vi "运维调试_质控单元.vi"() -> ()   [LabVIEW 2016, in "质控单元.lvlib"]
uses:
  <vilib>/Utility/miscctls.llb/LVPointTypeDef.ctl
  <vilib>/Utility/config.llb/Read Key (I32).vi
  <vilib>/Utility/config.llb/Read Key (Boolean).vi
  <vilib>/Utility/config.llb/Read Key (U32).vi
  <vilib>/Utility/config.llb/Write Key (I32).vi
  <vilib>/Utility/config.llb/Write Key (Boolean).vi
  <vilib>/Utility/config.llb/NI_LVConfig.lvlib
panel:
  out "CODCr母液浓度":dbl caption="加标母液浓度" format="%.2f"
  out "CODCr加标水杯定容体积":dbl caption="加标水杯定容体积" format="%.2f"
  out "CODCr检出限":dbl caption="检出限" format="%.2f"
  out "CODCr量程":dbl caption="量程" format="%.2f"
  out "COD母液浓度":dbl caption="加标母液浓度" format="%.2f"
  out "COD加标水杯定容体积":dbl caption="加标水杯定容体积" format="%.2f"
  out "COD检出限":dbl caption="检出限" format="%.2f"
  out "COD量程":dbl caption="量程" format="%.2f"
  out "总氮母液浓度":dbl caption="加标母液浓度" format="%.3f"
  out "总氮加标水杯定容体积":dbl caption="加标水杯定容体积" format="%.2f"
  out "总氮检出限":dbl caption="检出限" format="%.3f"
  out "总氮量程":dbl caption="量程" format="%.2f"
  out "总磷母液浓度":dbl caption="加标母液浓度" format="%.3f"
  out "总磷加标水杯定容体积":dbl caption="加标水杯定容体积" format="%.2f"
  out "总磷检出限":dbl caption="检出限" format="%.3f"
  out "总磷量程":dbl caption="量程" format="%.2f"
  out "氨氮母液浓度":dbl caption="加标母液浓度" format="%.3f"
  out "氨氮加标水杯定容体积":dbl caption="加标水杯定容体积" format="%.2f"
  out "氨氮检出限":dbl caption="检出限" format="%.3f"
  out "氨氮量程":dbl caption="量程" format="%.2f"
  in  "释放串口":bool
  in  "打开串口":bool
  out "CODCr质控流程中":bool
  out "CODMn质控流程中":bool
  out "总磷质控流程中":bool
  out "总氮质控流程中":bool
  out "氨氮质控流程中":bool
  out "CODCr通讯":bool
  out "CODMn通讯":bool
  out "总磷总氮通讯":bool
  out "氨氮通讯":bool
  out "CODCr传感器状态显示":bool
  out "CODCr超时报警":bool
  out "CODMn超时报警":bool
  out "总磷总氮超时报警":bool
  out "氨氮进样超时报警":bool
  out "CODMn传感器状态显示":bool
  out "总磷总氮传感器状态显示":bool
  out "氨氮传感器状态显示":bool
  out "CODCr流程中断报警":bool
  out "总磷总氮流程中断报警":bool
  out "CODMn流程中断报警":bool
  out "氨氮流程中断报警":bool
  in  "手动调试":bool
  in  "报警清除":bool
  in  "查看":bool
  in  "停止测量":bool
  in  "加标回收":bool
  in  "平行样测试":bool
  in  "CODCr量程选择":enum32{"H", "L", "AUTO"}(ring)
  in  "CODCr选择":bool
  out "CODCr加标回收率":dbl caption="加标回收率" format="%.2f"
  out "CODCr加标体积":dbl caption="加标体积" format="%.3f"
  out "CODCr加标后水样浓度":dbl caption="加标后水样浓度" format="%.2f"
  out "CODCr加标前水样浓度":dbl caption="加标前水样浓度" format="%.2f"
  out "CODCr状态":u16(ring) caption="状态" items=["待机", "润洗", "进样", "等待取液", "排液"]
  out "质控流程中":bool
  in  "CODMn量程选择":enum32{"H", "L", "AUTO"}(ring)
  in  "总磷量程选择":enum32{"H", "L", "AUTO"}(ring)=enum."AUTO"
  in  "总氮量程选择":enum32{"H", "L", "AUTO"}(ring)=enum."AUTO"
  in  "氨氮量程选择":enum32{"H", "L", "AUTO"}(ring)=enum."AUTO"
  in  "CODMn选择":bool
  in  "总磷总氮模块选择":bool
  in  "氨氮模块":bool
  in  "背隙补偿步数 3":i32 min=0 max=2000
  in  "背隙补偿步数 2":i32 min=0 max=2000
  in  "背隙补偿步数":i32 min=0 max=2000
  out "总氮加标回收率":dbl caption="加标回收率" format="%.2f"
  out "总氮加标体积":dbl caption="加标体积" format="%.3f"
  out "总氮加标后水样浓度":dbl caption="加标后水样浓度" format="%.3f"
  out "总氮加标前水样浓度":dbl caption="加标前水样浓度" format="%.3f"
  out "总氮状态":u16(ring) caption="状态" items=["待机", "润洗", "进样", "等待取液", "排液"]
  in  "返回":bool
  out "COD加标回收率":dbl caption="加标回收率" format="%.2f"
  out "COD加标体积":dbl caption="加标体积" format="%.3f"
  out "COD加标后水样浓度":dbl caption="加标后水样浓度" format="%.2f"
  out "COD加标前水样浓度":dbl caption="加标前水样浓度" format="%.2f"
  out "CODMn状态":u16(ring) caption="状态" items=["待机", "润洗", "进样", "等待取液", "排液"]
  out "总磷加标回收率":dbl caption="加标回收率" format="%.2f"
  out "总磷加标体积":dbl caption="加标体积" format="%.3f"
  out "总磷加标后水样浓度":dbl caption="加标后水样浓度" format="%.3f"
  out "总磷加标前水样浓度":dbl caption="加标前水样浓度" format="%.3f"
  out "总磷状态":u16(ring) caption="状态" items=["待机", "润洗", "进样", "等待取液", "排液"]
  out "氨氮加标回收率":dbl caption="加标回收率" format="%.2f"
  out "氨氮加标体积":dbl caption="加标体积" format="%.3f"
  out "氨氮加标后水样浓度":dbl caption="加标后水样浓度" format="%.3f"
  out "氨氮加标前水样浓度":dbl caption="加标前水样浓度" format="%.3f"
  out "氨氮状态":u16(ring) caption="状态" items=["待机", "润洗", "进样", "等待取液", "排液"]
  # "氨氮"
  # "总磷"
  # "总氮"
  # "CODMn"
  # "CODCr"
  # "参数配置区"
  # "2000步等于1mL\n100步等于0.05mL\n20步等于0.01mL\n2步等于0.001mL\n（初始默认100步）"
  # "CODCr质控参数"
  # "mg/L"
  # "mL"
  # "mg/L"
  # "mg/L"
  # "CODMn质控参数"
  # "mg/L"
  # "mL"
  # "mg/L"
  # "mg/L"
  # "总氮质控参数"
  # "mg/L"
  # "mL"
  # "mg/L"
  # "mg/L"
  # "总磷质控参数"
  # "mg/L"
  # "mL"
  # "mg/L"
  # "mg/L"
  # "氨氮质控参数"
  # "mg/L"
  # "mL"
  # "mg/L"
  # "mg/L"
  # "%"
  # "mL"
  # "mg/L"
  # "mg/L"
  # "%"
  # "mL"
  # "mg/L"
  # "mg/L"
  # "%"
  # "mL"
  # "mg/L"
  # "mg/L"
  # "%"
  # "mL"
  # "mg/L"
  # "mg/L"
  # "%"
  # "mL"
  # "mg/L"
  # "mg/L"
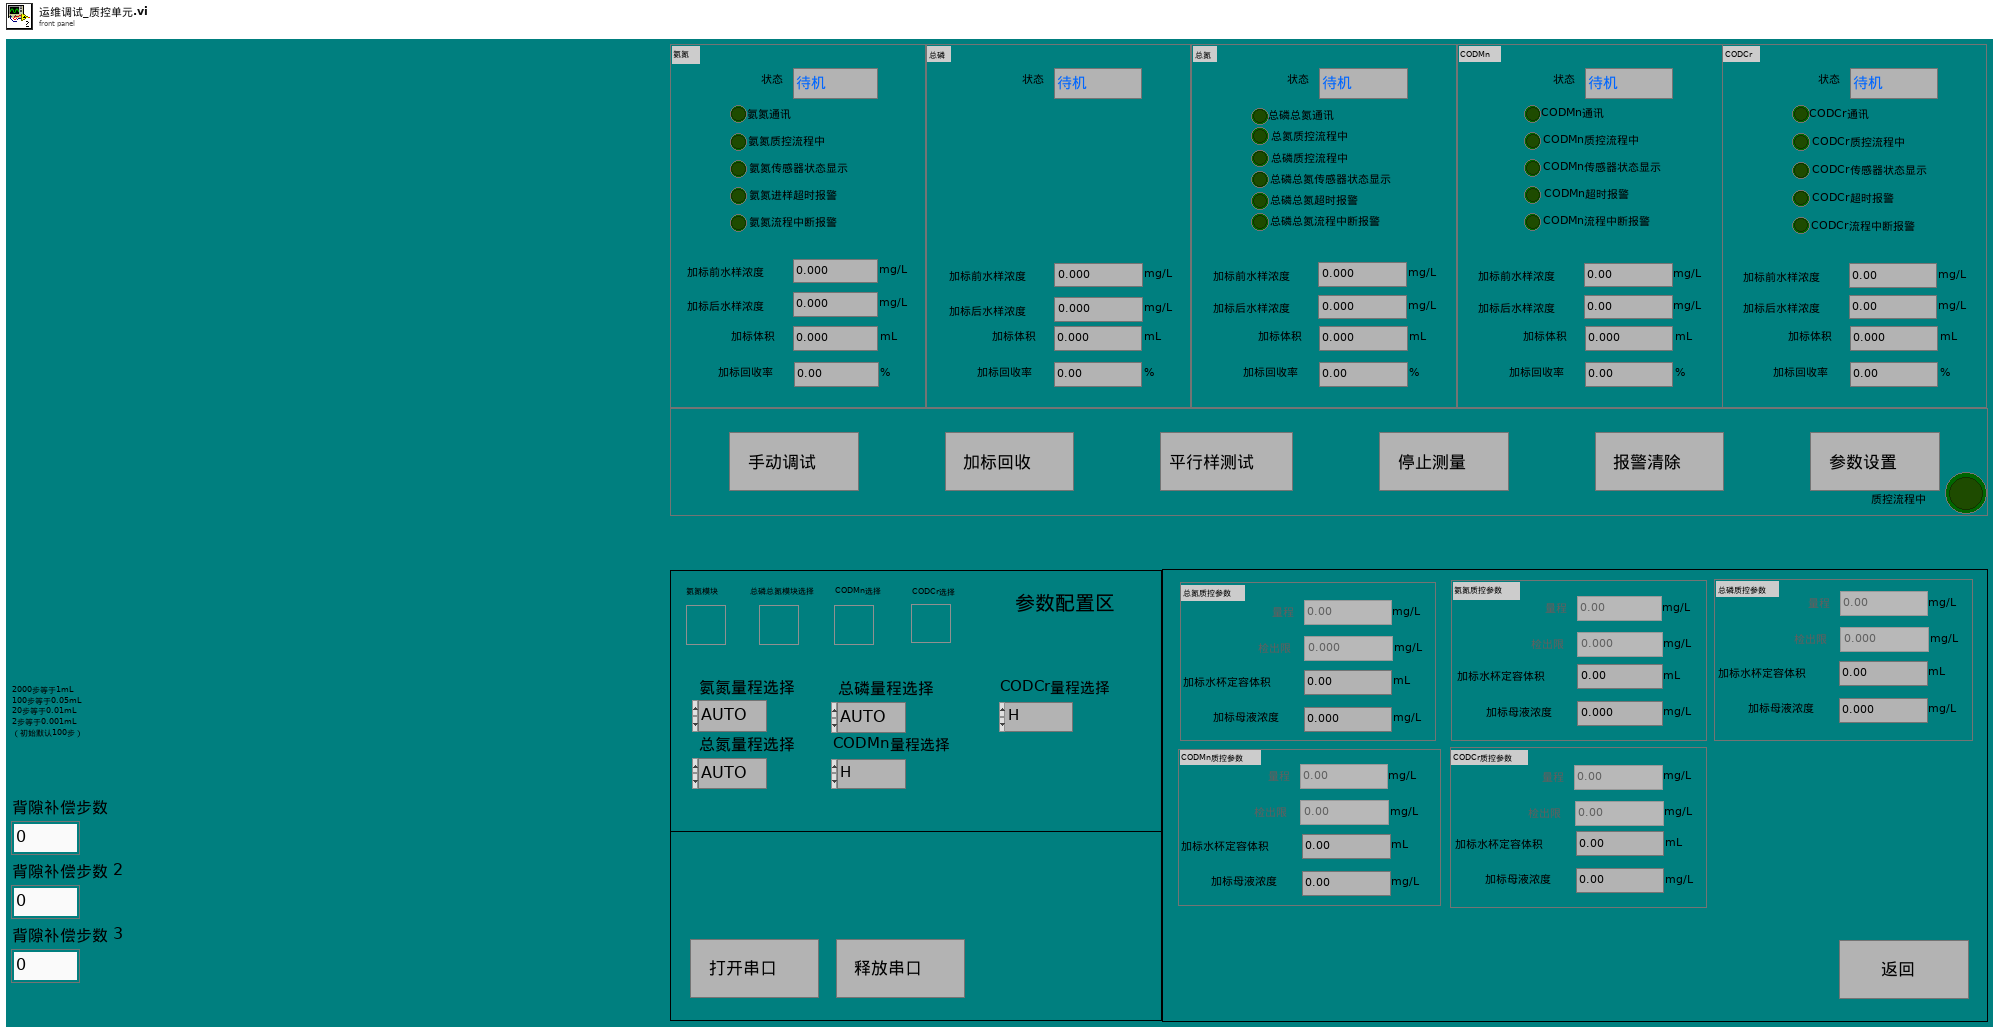
[diagram p1: front panel]
types:
  T1 = typedef "LVPointTypeDef.ctl" = cluster{"Horizontal":i16, "Vertical":i16}
  T2 = typedef "NI_LVConfig.lvlib/Config Data RefNum.ctl" = refnum<k1>
  T3 = cluster{"量程":dbl, "检出限":dbl, "加标前水样浓度":dbl, "加标后水样浓度":dbl, "加标水杯定容体积":dbl, "加标母液浓度":dbl, "加标体积":dbl, "加标回收率":dbl}
  T4 = enum8{"Enabled", "Disabled", "Disabled and Grayed Out"}
  T5 = cluster{"是否启用仪器":bool, "CODMn":cluster{"启动测量模式":cluster{"测量模式":enum16{"水样测量", "标样核查", "加标回收", "平行样", "校零", "校标"}}, "确定按钮":bool}, "启动模块":cluster{"氨氮":bool, "总磷":bool, "总氮":bool, "CODMn":bool, "CODCr":bool}, "常规启动":bool, "直接启动":bool}
  T6 = cluster{"参数启用":cluster{"CODMn":bool, "总磷":bool, "总氮":bool, "氨氮":bool, "CODcr":bool}, "采配水是否启动":bool}
  T7 = cluster{"命令":string, cluster{"starting address":u16, "holding register value":u16}}
  T8 = cluster{"氨氮":bool, "总磷":bool, "总氮":bool, "CODMn":bool, "CODCr":bool}
  T9 = enum32{"Bad", "Idle", "Run top level", "Running"}
  T10 = cluster{"CODMn":bool, "总磷":bool, "总氮":bool, "氨氮":bool, "CODCr":bool}
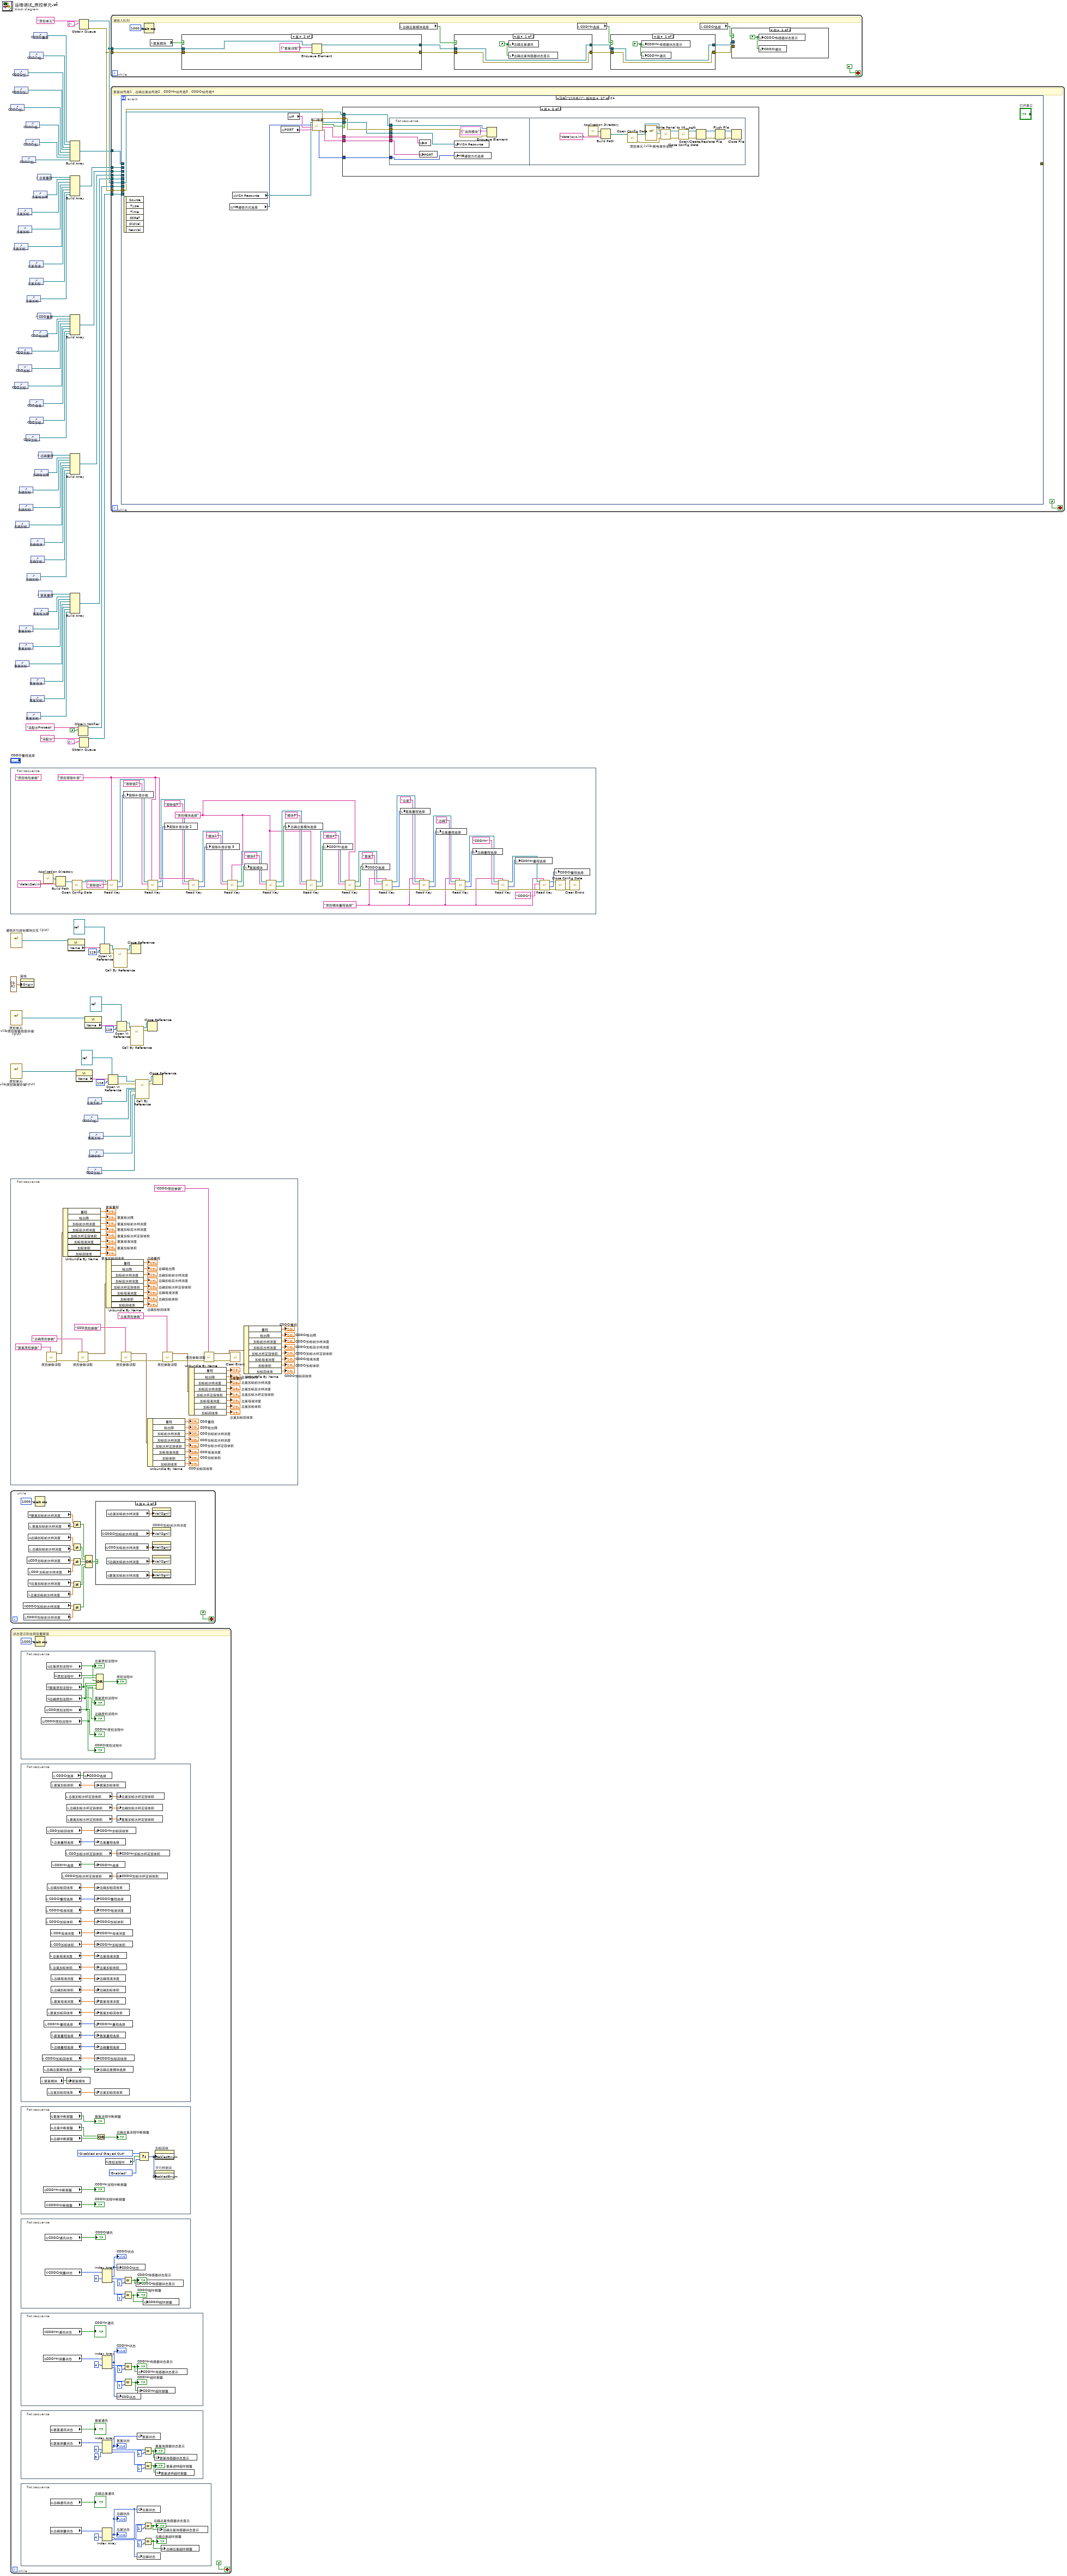
[diagram p0: block diagram]
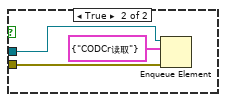
[diagram p2: hidden frame]
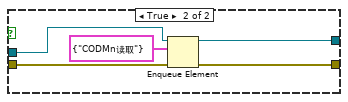
[diagram p3: hidden frame]
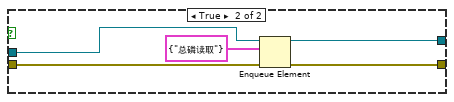
[diagram p4: hidden frame]
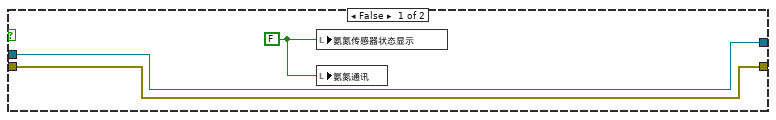
[diagram p5: hidden frame]
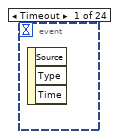
[diagram p7: hidden frame]
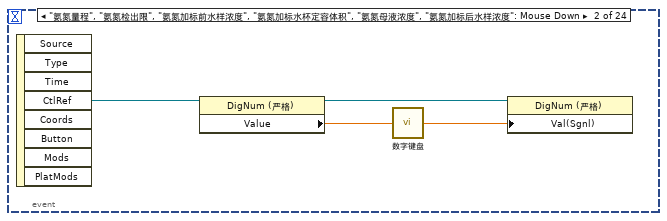
[diagram p8: hidden frame]
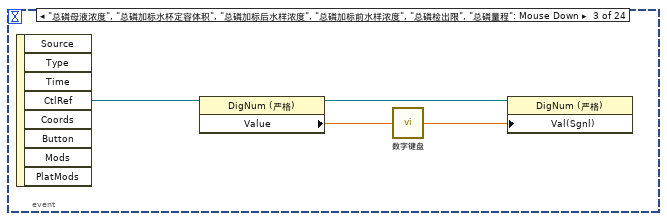
[diagram p9: hidden frame]
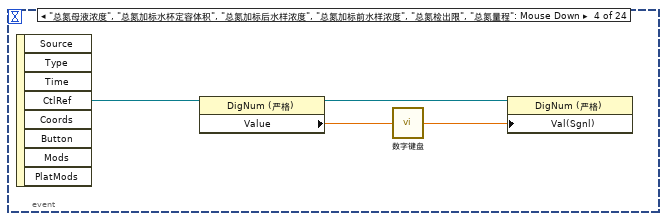
[diagram p10: hidden frame]
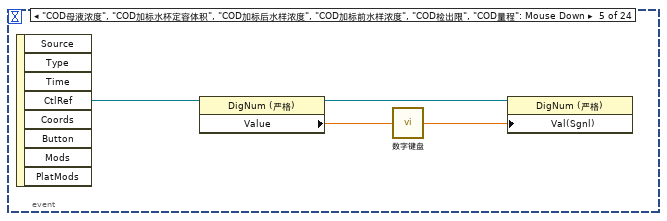
[diagram p11: hidden frame]
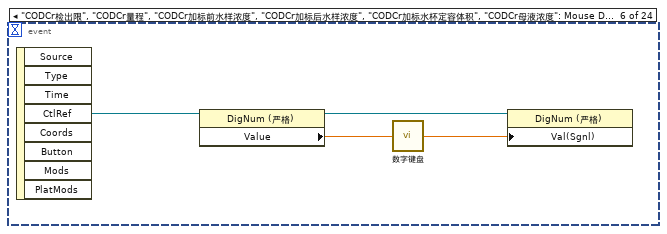
[diagram p12: hidden frame]
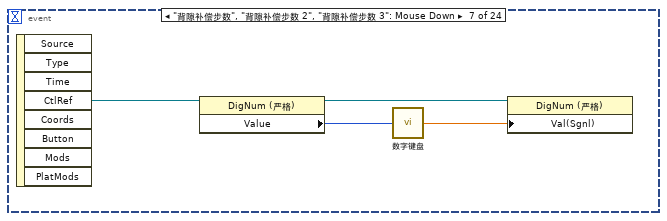
[diagram p13: hidden frame]
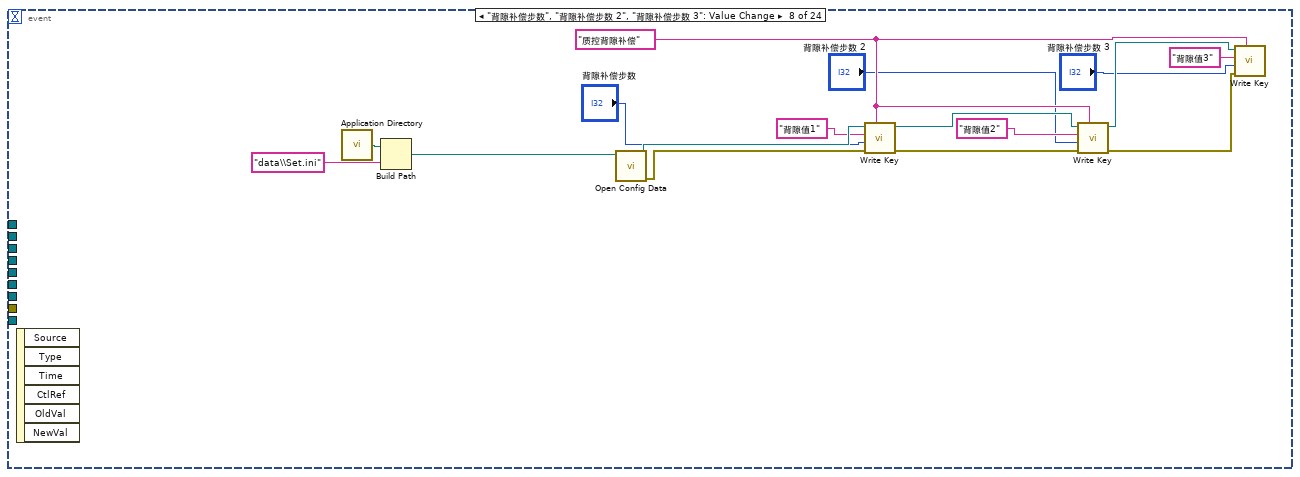
[diagram p14: hidden frame]
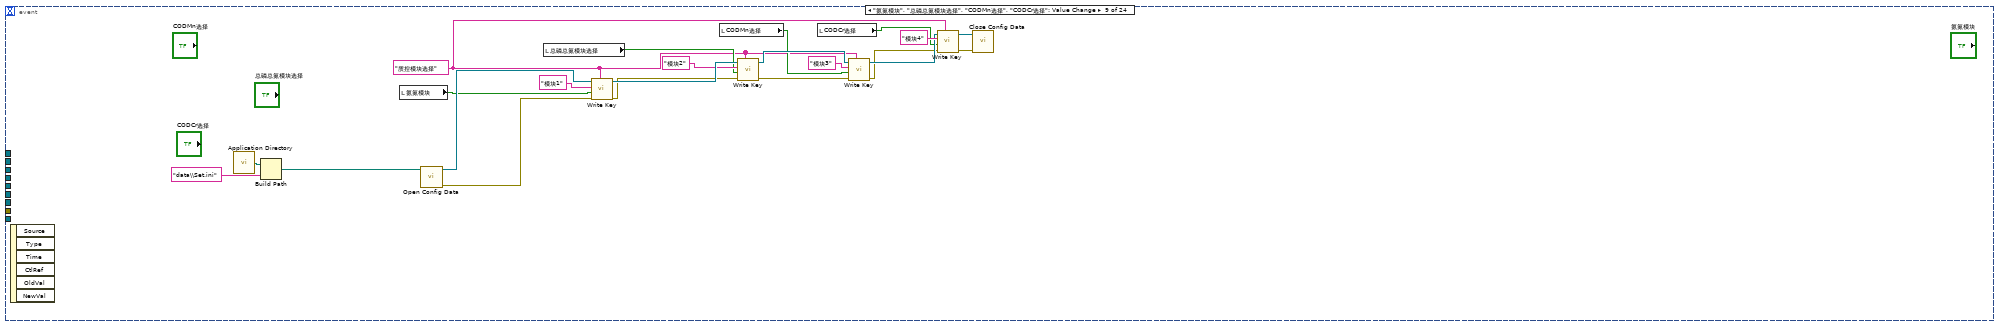
[diagram p15: hidden frame]
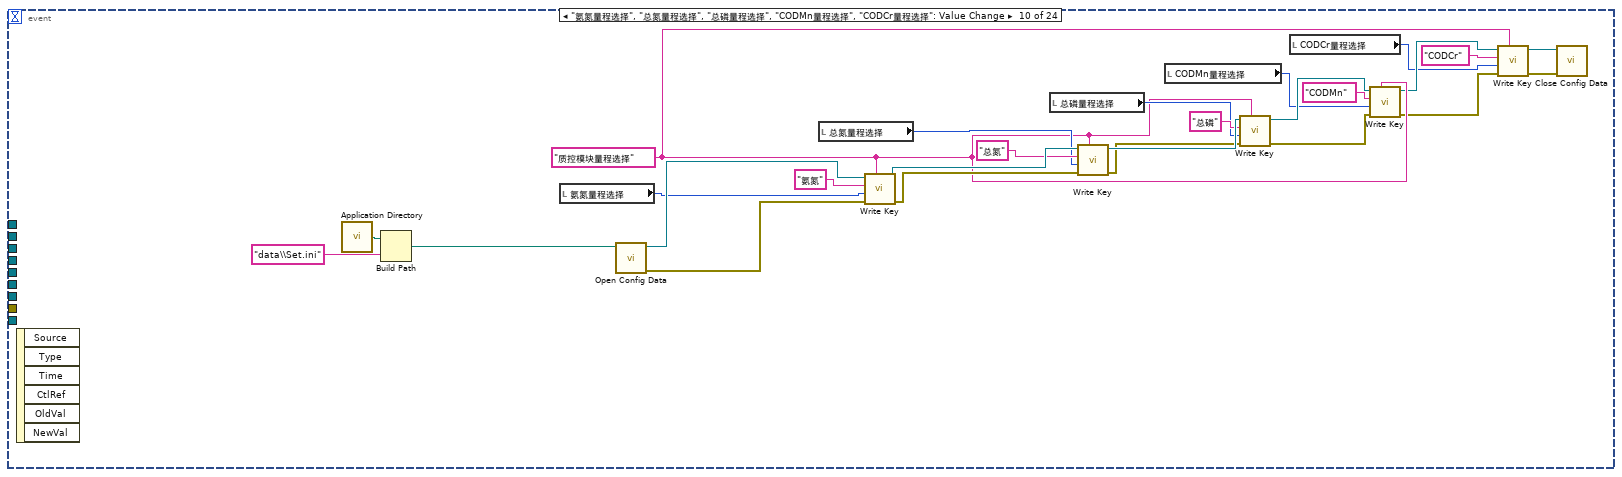
[diagram p16: hidden frame]
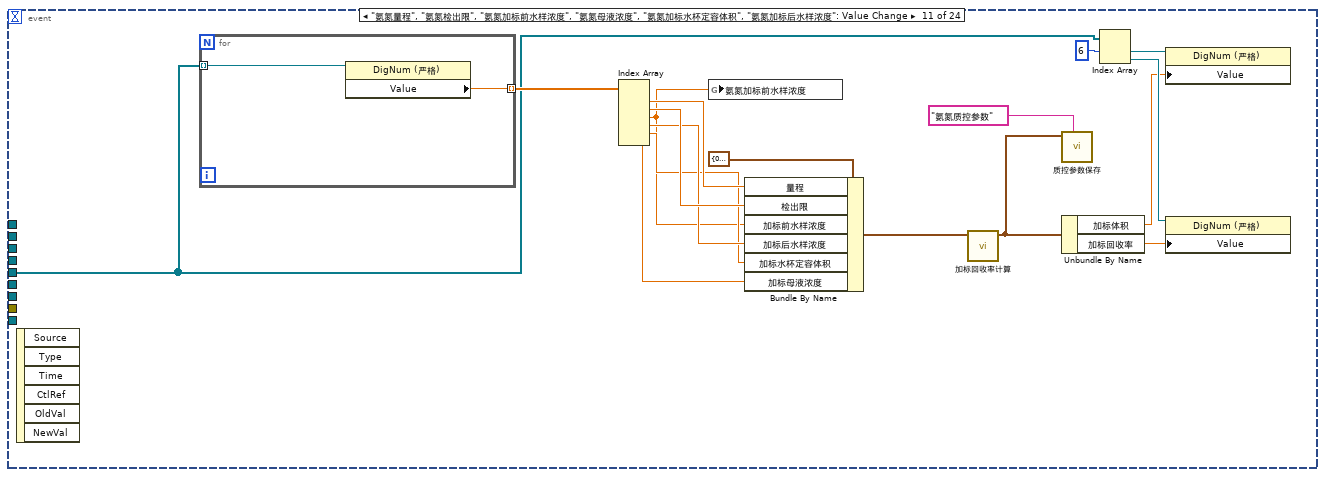
[diagram p17: hidden frame]
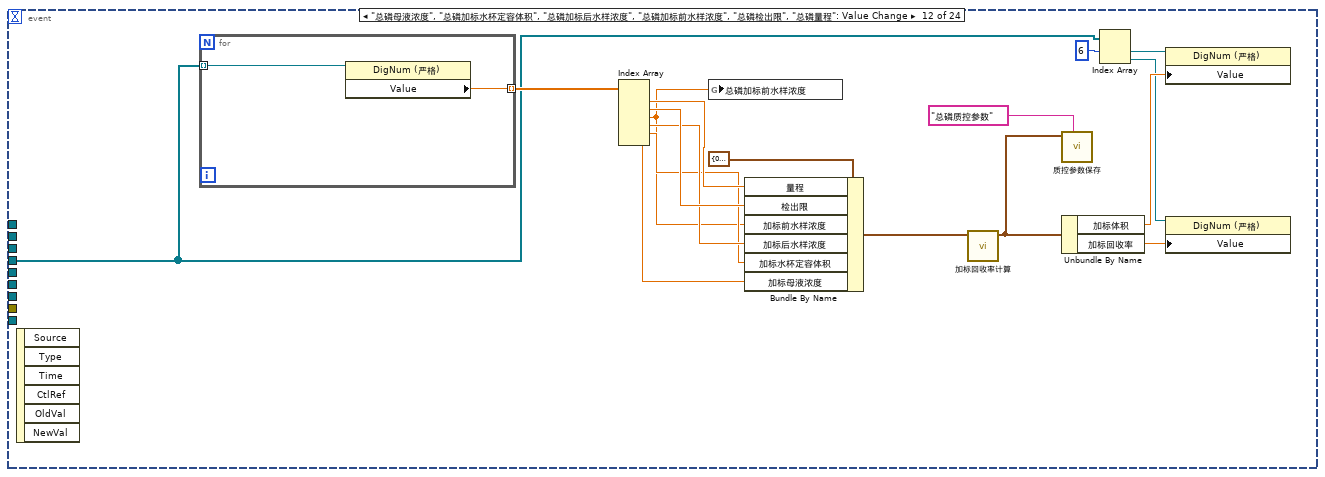
[diagram p18: hidden frame]
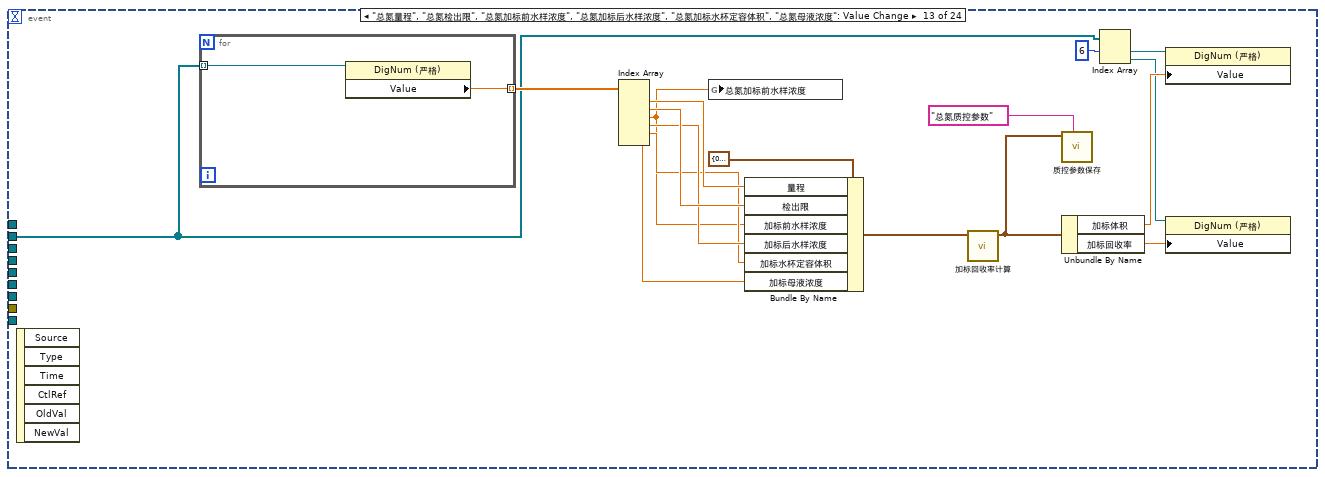
[diagram p19: hidden frame]
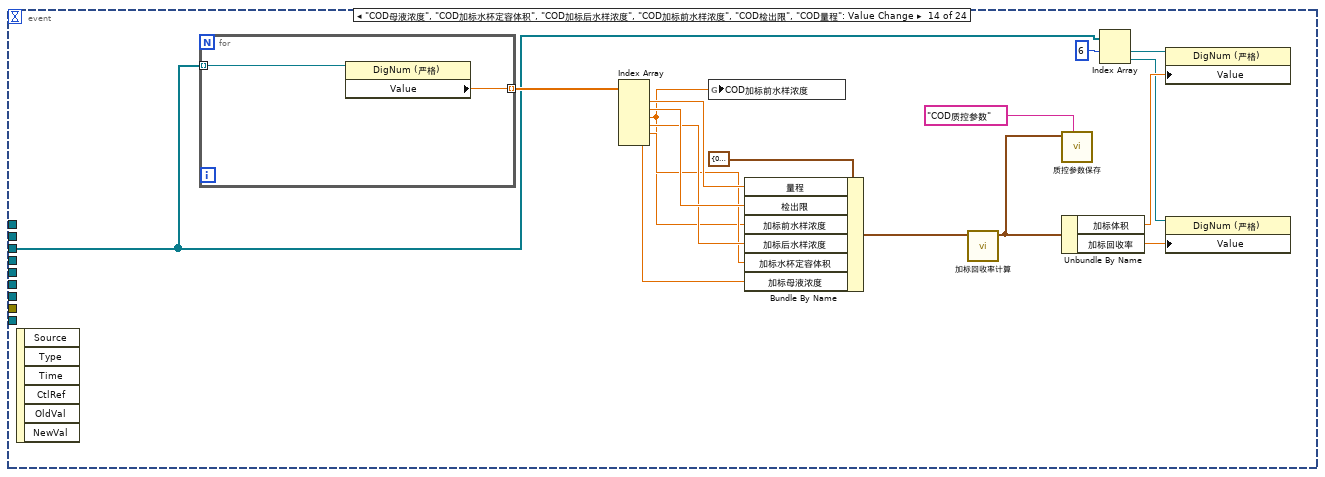
[diagram p20: hidden frame]
diagram:
  n1 = control-ref of="CODCr加标水杯定容体积"() -> (w38:refnum<vi>)
  n2 = flat-sequence {
    frame #0 {
      w100 = "质控模块量程选择" ("section")
      w92 = "质控模块选择" ("section")
      (unwired) "质控线性参数" ("section")
      w136 = "质控背隙补偿" ("section")
      n3 = call <vilib>:"Application Directory.vi"() -> ("Application Directory"=w142:path)
      n4 = Build Path(base path=w142, name or relative path="data\\Set.ini" ("名称或相对路径")) -> (appended path=w140:path)
      n5 = call <vilib>:"Open Config Data.vi"("configuration file path"=w140) -> ("error out"=w138:errorcluster, "refnum"=w139:T2)  [unwired: 8 in, 1 out]
      n6 = call-poly <vilib>:"Read Key.vi"("section"=w136, "error in (no error)"=w138, "key"="背隙值1", "refnum"=w139) -> ("error out"=w133:errorcluster, "value"=w128:i32, "refnum out"=w135:T2)  [unwired: 4 in, 1 out]
      n7 = local write "背隙补偿步数"(w128) -> ()
      n8 = call-poly <vilib>:"Read Key.vi"("section"=w136, "error in (no error)"=w133, "key"="背隙值2", "refnum"=w135) -> ("error out"=w131:errorcluster, "value"=w129:i32, "refnum out"=w132:T2)  [unwired: 4 in, 1 out]
      n9 = local write "背隙补偿步数 2"(w129) -> ()
      n10 = call-poly <vilib>:"Read Key.vi"("section"=w136, "error in (no error)"=w131, "key"="背隙值3", "refnum"=w132) -> ("error out"=w87:errorcluster, "value"=w127:i32, "refnum out"=w88:T2)  [unwired: 4 in, 1 out]
      n11 = local write "背隙补偿步数 3"(w127) -> ()
      n12 = call-poly <vilib>:"Read Key.vi"("section"=w92, "error in (no error)"=w87, "key"="模块1" ("section"), "refnum"=w88) -> ("error out"=w125:errorcluster, "value"=w117:bool, "refnum out"=w126:T2)  [unwired: 4 in, 1 out]
      n13 = local write "氨氮模块"(w117) -> ()
      n14 = call-poly <vilib>:"Read Key.vi"("section"=w92, "error in (no error)"=w125, "key"="模块2" ("section"), "refnum"=w126) -> ("error out"=w123:errorcluster, "value"=w118:bool, "refnum out"=w124:T2)  [unwired: 4 in, 1 out]
      n15 = local write "总磷总氮模块选择"(w118) -> ()
      n16 = call-poly <vilib>:"Read Key.vi"("section"=w92, "error in (no error)"=w123, "key"="模块3" ("section"), "refnum"=w124) -> ("error out"=w94:errorcluster, "value"=w119:bool, "refnum out"=w95:T2)  [unwired: 4 in, 1 out]
      n17 = local write "CODMn选择"(w119) -> ()
      n18 = call-poly <vilib>:"Read Key.vi"("section"=w92, "error in (no error)"=w94, "key"="模块4", "refnum"=w95) -> ("error out"=w90:errorcluster, "value"=w89:bool, "refnum out"=w91:T2)  [unwired: 4 in, 1 out]
      n19 = local write "CODCr选择"(w89) -> ()
      n20 = call-poly <vilib>:"Read Key.vi"("section"=w100, "error in (no error)"=w90, "key"="氨氮" ("section"), "refnum"=w91) -> ("error out"=w115:errorcluster, "value"=w106:u32, "refnum out"=w116:T2)  [unwired: 4 in, 1 out]
      n21 = local write "氨氮量程选择"(w106) -> ()
      n22 = call-poly <vilib>:"Read Key.vi"("section"=w100, "error in (no error)"=w115, "key"="总氮" ("section"), "refnum"=w116) -> ("error out"=w113:errorcluster, "value"=w105:u32, "refnum out"=w114:T2)  [unwired: 4 in, 1 out]
      n23 = local write "总氮量程选择"(w105) -> ()
      n24 = call-poly <vilib>:"Read Key.vi"("section"=w100, "error in (no error)"=w113, "key"="总磷" ("section"), "refnum"=w114) -> ("error out"=w111:errorcluster, "value"=w104:u32, "refnum out"=w112:T2)  [unwired: 4 in, 1 out]
      n25 = local write "总磷量程选择"(w104) -> ()
      n26 = call-poly <vilib>:"Read Key.vi"("section"=w100, "error in (no error)"=w111, "key"="CODMn" ("section"), "refnum"=w112) -> ("error out"=w101:errorcluster, "value"=w103:u32, "refnum out"=w102:T2)  [unwired: 4 in, 1 out]
      n27 = local write "CODMn量程选择"(w103) -> ()
      n28 = call-poly <vilib>:"Read Key.vi"("section"=w100, "error in (no error)"=w101, "key"="CODCr" ("section"), "refnum"=w102) -> ("error out"=w97:errorcluster, "value"=w98:u32, "refnum out"=w96:T2)  [unwired: 4 in, 1 out]
      n29 = local write "CODCr量程选择"(w98) -> ()
      n30 = call <vilib>:"Close Config Data.vi"("error in (no error)"=w97, "refnum"=w96) -> ("error out"=w86:errorcluster)  [unwired: 8 in, 1 out]
      n31 = call <vilib>:"Clear Errors.vi"("error in (no error)"=w86) -> ()  [unwired: 5 in, 2 out]
    }
  }
  n32 = vi-ref "通信并与其他模块交互 (子VI).vi"() -> (w26:refnum<vi>)
  n33 = vi-ref "质控单元.lvlib:质控报警信息存储 (子VI).vi"() -> (w21:refnum<vi>)
  n34 = vi-ref "质控单元.lvlib:质控数据存储(子VI).vi"() -> (w6:refnum<vi>)
  n35 = flat-sequence {
    frame #0 {
      n36 = call "质控参数读取.vi"("section"="氨氮质控参数") -> ("error out"=w177:errorcluster, "参数"=w196:T3)  [unwired: 9 in]
      n37 = Unbundle By Name(w196) -> ("量程"=→"氨氮量程":dbl, "检出限"=→"氨氮检出限":dbl, "加标前水样浓度"=→"氨氮加标前水样浓度":dbl, "加标后水样浓度"=→"氨氮加标后水样浓度":dbl, "加标水杯定容体积"=→"氨氮加标水杯定容体积":dbl, "加标母液浓度"=→"氨氮母液浓度":dbl, "加标体积"=→"氨氮加标体积":dbl, "加标回收率"=→"氨氮加标回收率":dbl)
      n38 = call "质控参数读取.vi"("section"="总磷质控参数", "error in (no error)"=w177) -> ("error out"=w174:errorcluster, "参数"=w186:T3)  [unwired: 8 in]
      n39 = Unbundle By Name(w186) -> ("量程"=→"总磷量程":dbl, "检出限"=→"总磷检出限":dbl, "加标前水样浓度"=→"总磷加标前水样浓度":dbl, "加标后水样浓度"=→"总磷加标后水样浓度":dbl, "加标水杯定容体积"=→"总磷加标水杯定容体积":dbl, "加标母液浓度"=→"总磷母液浓度":dbl, "加标体积"=→"总磷加标体积":dbl, "加标回收率"=→"总磷加标回收率":dbl)
      n40 = call "质控参数读取.vi"("section"="COD质控参数", "error in (no error)"=w174) -> ("error out"=w164:errorcluster, "参数"=w176:T3)  [unwired: 8 in]
      n41 = Unbundle By Name(w176) -> ("量程"=→"COD量程":dbl, "检出限"=→"COD检出限":dbl, "加标前水样浓度"=→"COD加标前水样浓度":dbl, "加标后水样浓度"=→"COD加标后水样浓度":dbl, "加标水杯定容体积"=→"COD加标水杯定容体积":dbl, "加标母液浓度"=→"COD母液浓度":dbl, "加标体积"=→"COD加标体积":dbl, "加标回收率"=→"COD加标回收率":dbl)
      n42 = call "质控参数读取.vi"("section"="总氮质控参数", "error in (no error)"=w164) -> ("error out"=w152:errorcluster, "参数"=w163:T3)  [unwired: 8 in]
      n43 = Unbundle By Name(w163) -> ("量程"=→"总氮量程":dbl, "检出限"=→"总氮检出限":dbl, "加标前水样浓度"=→"总氮加标前水样浓度":dbl, "加标后水样浓度"=→"总氮加标后水样浓度":dbl, "加标水杯定容体积"=→"总氮加标水杯定容体积":dbl, "加标母液浓度"=→"总氮母液浓度":dbl, "加标体积"=→"总氮加标体积":dbl, "加标回收率"=→"总氮加标回收率":dbl)
      n44 = call "质控参数读取.vi"("section"="CODCr质控参数", "error in (no error)"=w152) -> ("error out"=w143:errorcluster, "参数"=w153:T3)  [unwired: 8 in]
      n45 = call <vilib>:"Clear Errors.vi"("error in (no error)"=w143) -> ()  [unwired: 5 in, 2 out]
      n46 = Unbundle By Name(w153) -> ("量程"=→"CODCr量程":dbl, "检出限"=→"CODCr检出限":dbl, "加标前水样浓度"=→"CODCr加标前水样浓度":dbl, "加标后水样浓度"=→"CODCr加标后水样浓度":dbl, "加标水杯定容体积"=→"CODCr加标水杯定容体积":dbl, "加标母液浓度"=→"CODCr母液浓度":dbl, "加标体积"=→"CODCr加标体积":dbl, "加标回收率"=→"CODCr加标回收率":dbl)
    }
  }
  n47 = while {
    stop <- FALSE stop-if-true
    n48 = global read "水样浓度全局.vi" "CODCr加标前水样浓度"() -> (w200:dbl)
    n49 = local read "CODCr加标前水样浓度"() -> (w199:dbl)
    n50 = global read "水样浓度全局.vi" "COD加标前水样浓度"() -> (w209:dbl)
    n51 = local read "总氮加标前水样浓度"() -> (w203:dbl)
    n52 = global read "水样浓度全局.vi" "氨氮加标前水样浓度"() -> (w213:dbl)
    n53 = global read "水样浓度全局.vi" "总磷加标前水样浓度"() -> (w211:dbl)
    n54 = local read "COD加标前水样浓度"() -> (w208:dbl)
    n55 = global read "水样浓度全局.vi" "总氮加标前水样浓度"() -> (w202:dbl)
    n56 = local read "氨氮加标前水样浓度"() -> (w212:dbl)
    n57 = local read "总磷加标前水样浓度"() -> (w210:dbl)
    n58 = Wait (ms)(milliseconds to wait=u32 1000 ("等待时间（毫秒）")) -> ()  [unwired: 1 out]
    n59 = Not Equal?(x=w213, y=w212) -> (x != y?=w207:bool)
    n60 = Not Equal?(x=w211, y=w210) -> (x != y?=w205:bool)
    n61 = Not Equal?(x=w209, y=w208) -> (x != y?=w204:bool)
    n62 = Not Equal?(x=w202, y=w203) -> (x != y?=w201:bool)
    n63 = Not Equal?(x=w200, y=w199) -> (x != y?=w198:bool)
    n64 = Compound Arithmetic op=OR ("复合运算")(w207, w205, w204, w201, w198) -> (w206:bool)
    n65 = case shown="真" w206 {
      frame False {
      }
      frame True {
        n66 = global read "水样浓度全局.vi" "CODCr加标前水样浓度"() -> (w216:dbl)
        n67 = global read "水样浓度全局.vi" "COD加标前水样浓度"() -> (w218:dbl)
        n68 = global read "水样浓度全局.vi" "总氮加标前水样浓度"() -> (w217:dbl)
        n69 = global read "水样浓度全局.vi" "总磷加标前水样浓度"() -> (w219:dbl)
        n70 = global read "水样浓度全局.vi" "氨氮加标前水样浓度"() -> (w220:dbl)
        n71 = property on="总氮加标前水样浓度" class="DigNum (严格)"("Val(Sgnl)"=w217) -> ()  [unwired: 2 in, 2 out]
        n72 = property on="CODCr加标前水样浓度" class="DigNum (严格)"("Val(Sgnl)"=w216) -> ()  [unwired: 2 in, 2 out]
        n73 = property on="COD加标前水样浓度" class="DigNum (严格)"("Val(Sgnl)"=w218) -> ()  [unwired: 2 in, 2 out]
        n74 = property on="总磷加标前水样浓度" class="DigNum (严格)"("Val(Sgnl)"=w219) -> ()  [unwired: 2 in, 2 out]
        n75 = property on="氨氮加标前水样浓度" class="DigNum (严格)"("Val(Sgnl)"=w220) -> ()  [unwired: 2 in, 2 out]
      }
    }
  }
  n76 = while {
    stop <- FALSE stop-if-true
    # "状态显示和全局变量赋值"
    n77 = flat-sequence {
      frame #0 {
        n78 = global read "质控测完标志全局 1.vi" "CODCr质控流程中"() -> (w303:bool)
        "CODCr质控流程中" <- w303
        n79 = global read "质控测完标志全局 1.vi" "COD质控流程中"() -> (w304:bool)
        "CODMn质控流程中" <- w304
        n80 = global read "质控测完标志全局 1.vi" "总氮质控流程中"() -> (w306:bool)
        "总氮质控流程中" <- w306
        n81 = global read "质控测完标志全局 1.vi" "氨氮质控流程中"() -> (w307:bool)
        "氨氮质控流程中" <- w307
        n82 = global read "质控测完标志全局 1.vi" "总磷质控流程中"() -> (w305:bool)
        "总磷质控流程中" <- w305
        n83 = global read "质控测完标志全局 1.vi" "质控流程中"() -> (w309:bool)
        n84 = Compound Arithmetic op=OR ("复合运算")(w309, w307, w306, w305, w304, w303) -> (→"质控流程中":bool)
      }
    }
    n85 = flat-sequence {
      frame #0 {
        n86 = local read "氨氮模块"() -> (w297:bool)
        n87 = local read "CODCr加标回收率"() -> (w278:dbl)
        n88 = local read "总磷总氮模块选择"() -> (w296:bool)
        n89 = local read "CODMn量程选择"() -> (w301:enum32{"H", "L", "AUTO"})
        n90 = local read "CODCr量程选择"() -> (w302:enum32{"H", "L", "AUTO"})
        n91 = local read "CODCr母液浓度"() -> (w279:dbl)
        n92 = local read "CODCr加标体积"() -> (w289:dbl)
        n93 = local read "COD加标回收率"() -> (w277:dbl)
        n94 = local read "总磷加标回收率"() -> (w275:dbl)
        n95 = local read "氨氮加标回收率"() -> (w274:dbl)
        n96 = local read "总氮加标回收率"() -> (w276:dbl)
        n97 = local read "总氮母液浓度"() -> (w281:dbl)
        n98 = local read "总氮加标体积"() -> (w291:dbl)
        n99 = local read "COD母液浓度"() -> (w280:dbl)
        n100 = local read "COD加标体积"() -> (w290:dbl)
        n101 = local read "氨氮加标体积"() -> (w293:dbl)
        n102 = local read "总氮量程选择"() -> (w299:enum32{"H", "L", "AUTO"})
        n103 = local read "总磷母液浓度"() -> (w282:dbl)
        n104 = local read "总磷加标体积"() -> (w292:dbl)
        n105 = local read "氨氮母液浓度"() -> (w283:dbl)
        n106 = local read "氨氮量程选择"() -> (w300:enum32{"H", "L", "AUTO"})
        n107 = local read "总磷量程选择"() -> (w298:enum32{"H", "L", "AUTO"})
        n108 = local read "CODMn选择"() -> (w295:bool)
        n109 = local read "CODCr选择"() -> (w294:bool)
        n110 = local read "CODCr加标水杯定容体积"() -> (w288:dbl)
        n111 = local read "总氮加标水杯定容体积"() -> (w286:dbl)
        n112 = local read "COD加标水杯定容体积"() -> (w287:dbl)
        n113 = local read "总磷加标水杯定容体积"() -> (w285:dbl)
        n114 = local read "氨氮加标水杯定容体积"() -> (w284:dbl)
        n115 = global write "断电保存全局.vi" "氨氮模块"(w297) -> ()
        n116 = global write "断电保存全局.vi" "CODCr选择"(w294) -> ()
        n117 = global write "加标回收状态全局变量.vi" "氨氮加标体积"(w293) -> ()
        n118 = global write "加标回收状态全局变量.vi" "CODMn加标回收率"(w277) -> ()
        n119 = global write "断电保存全局.vi" "总氮量程选择"(w299) -> ()
        n120 = global write "断电保存全局.vi" "CODMn选择"(w295) -> ()
        n121 = global write "加标回收状态全局变量.vi" "总磷加标回收率"(w275) -> ()
        n122 = global write "断电保存全局.vi" "CODCr量程选择"(w302) -> ()
        n123 = global write "加标回收状态全局变量.vi" "CODCr母液浓度"(w279) -> ()
        n124 = global write "加标回收状态全局变量.vi" "CODCr加标体积"(w289) -> ()
        n125 = global write "加标回收状态全局变量.vi" "CODMn母液浓度"(w280) -> ()
        n126 = global write "加标回收状态全局变量.vi" "CODMn加标体积"(w290) -> ()
        n127 = global write "加标回收状态全局变量.vi" "总氮母液浓度"(w281) -> ()
        n128 = global write "加标回收状态全局变量.vi" "总氮加标体积"(w291) -> ()
        n129 = global write "加标回收状态全局变量.vi" "总磷母液浓度"(w282) -> ()
        n130 = global write "加标回收状态全局变量.vi" "总磷加标体积"(w292) -> ()
        n131 = global write "加标回收状态全局变量.vi" "氨氮母液浓度"(w283) -> ()
        n132 = global write "加标回收状态全局变量.vi" "氨氮加标回收率"(w274) -> ()
        n133 = global write "断电保存全局.vi" "CODMn量程选择"(w301) -> ()
        n134 = global write "断电保存全局.vi" "氨氮量程选择"(w300) -> ()
        n135 = global write "断电保存全局.vi" "总磷量程选择"(w298) -> ()
        n136 = global write "加标回收状态全局变量.vi" "CODCr加标回收率"(w278) -> ()
        n137 = global write "断电保存全局.vi" "总磷总氮模块选择"(w296) -> ()
        n138 = global write "加标回收状态全局变量.vi" "总氮加标回收率"(w276) -> ()
        n139 = global write "加标回收状态全局变量.vi" "总氮加标水杯定容体积"(w286) -> ()
        n140 = global write "加标回收状态全局变量.vi" "总磷加标水杯定容体积"(w285) -> ()
        n141 = global write "加标回收状态全局变量.vi" "氨氮加标水杯定容体积"(w284) -> ()
        n142 = global write "加标回收状态全局变量.vi" "CODMn加标水杯定容体积"(w287) -> ()
        n143 = global write "加标回收状态全局变量.vi" "CODCr加标水杯定容体积"(w288) -> ()
      }
    }
    n144 = flat-sequence {
      frame #0 {
        n145 = global read "质控中断报警全局.vi" "CODMn中断报警"() -> (→"CODMn流程中断报警":bool)
        n146 = global read "质控中断报警全局.vi" "CODCr中断报警"() -> (→"CODCr流程中断报警":bool)
        n147 = global read "质控中断报警全局.vi" "氨氮中断报警"() -> (→"氨氮流程中断报警":bool)
        n148 = global read "质控中断报警全局.vi" "总氮中断报警"() -> (w264:bool)
        n149 = global read "质控中断报警全局.vi" "总磷中断报警"() -> (w272:bool)
        n150 = Or(x=w264, y=w272) -> (x .or. y?=→"总磷总氮流程中断报警":bool)
        n151 = global read "质控测完标志全局 1.vi" "质控流程中"() -> (w269:bool)
        n152 = Select(t=T4."Disabled and Grayed Out" ("禁用"), s=w269, f=T4."Enabled") -> (s? t:f=w268:T4)
        n153 = property on="加标回收" class="Bool"("DisabledEnum"=w268) -> ()  [unwired: 2 in, 2 out]
        n154 = property on="平行样测试" class="Bool"("DisabledEnum"=w268) -> ()  [unwired: 2 in, 2 out]
      }
    }
    n155 = flat-sequence {
      frame #0 {
        n156 = global read "质控内部交互全局.vi" "CODCr通讯状态"() -> (→"CODCr通讯":bool)
        n157 = global read "质控内部交互全局.vi" "CODCr测量状态"() -> (w230:u16[])
        n158 = Index Array(array=w230, index #2=4 ("索引")) -> (element #1=w231:u16, element #2=w226:u16, element #3=w225:u16)  [unwired: 2 in]
        "CODCr状态" <- w231
        n159 = global write "加标回收状态全局变量.vi" "CODCr状态"(w231) -> ()
        n160 = Equal?(x=w226, y=u16 1) -> (x = y?=w223:bool)
        "CODCr传感器状态显示" <- w223
        n161 = Equal?(x=w225, y=u16 1) -> (x = y?=w224:bool)
        "CODCr超时报警" <- w224
        n162 = global write "质控中断报警全局.vi" "CODCr传感器状态显示"(w223) -> ()
        n163 = global write "质控中断报警全局.vi" "CODCr超时报警"(w224) -> ()
      }
    }
    n164 = flat-sequence {
      frame #0 {
        n165 = global read "质控内部交互全局.vi" "CODMn通讯状态"() -> (→"CODMn通讯":bool)
        n166 = global read "质控内部交互全局.vi" "CODMn测量状态"() -> (w238:u16[])
        n167 = Index Array(array=w238, index #2=4 ("索引")) -> (element #1=w241:u16, element #2=w239:u16, element #3=w235:u16)  [unwired: 2 in]
        "CODMn状态" <- w241
        n168 = global write "加标回收状态全局变量.vi" "COD状态"(w241) -> ()
        n169 = Equal?(x=w239, y=u16 1) -> (x = y?=w234:bool)
        "CODMn传感器状态显示" <- w234
        n170 = Equal?(x=w235, y=u16 1) -> (x = y?=w233:bool)
        "CODMn超时报警" <- w233
        n171 = global write "质控中断报警全局.vi" "CODMn超时报警"(w233) -> ()
        n172 = global write "质控中断报警全局.vi" "CODMn传感器状态显示"(w234) -> ()
      }
    }
    n173 = flat-sequence {
      frame #0 {
        n174 = global read "质控内部交互全局.vi" "氨氮通讯状态"() -> (→"氨氮通讯":bool)
        n175 = global read "质控内部交互全局.vi" "氨氮测量状态"() -> (w258:u16[])
        n176 = Index Array(array=w258, index #2=4 ("索引"), index #3=5 ("索引")) -> (element #1=w259:u16, element #2=w262:u16, element #3=w255:u16)  [unwired: 1 in]
        "氨氮状态" <- w259
        n177 = global write "加标回收状态全局变量.vi" "氨氮状态"(w259) -> ()
        n178 = Equal?(x=w262, y=u16 1) -> (x = y?=w254:bool)
        "氨氮传感器状态显示" <- w254
        n179 = Equal?(x=w255, y=u16 1) -> (x = y?=w253:bool)
        "氨氮进样超时报警" <- w253
        n180 = global write "质控中断报警全局.vi" "氨氮传感器状态显示"(w254) -> ()
        n181 = global write "质控中断报警全局.vi" "氨氮进样超时报警"(w253) -> ()
      }
    }
    n182 = flat-sequence {
      frame #0 {
        n183 = global read "质控内部交互全局.vi" "总磷通讯状态"() -> (→"总磷总氮通讯":bool)
        n184 = global read "质控内部交互全局.vi" "总磷测量状态"() -> (w248:u16[])
        n185 = Index Array(array=w248, index #2=4 ("索引")) -> (element #1=w249:u16, element #2=w250:u16, element #3=w245:u16)  [unwired: 2 in]
        "总氮状态" <- w249
        "总磷状态" <- w249
        n186 = global write "加标回收状态全局变量.vi" "总氮状态"(w249) -> ()
        n187 = global write "加标回收状态全局变量.vi" "总磷状态"(w249) -> ()
        n188 = Equal?(x=w250, y=u16 1) -> (x = y?=w244:bool)
        "总磷总氮传感器状态显示" <- w244
        n189 = Equal?(x=w245, y=u16 1) -> (x = y?=w243:bool)
        "总磷总氮超时报警" <- w243
        n190 = global write "质控中断报警全局.vi" "总磷总氮传感器状态显示"(w244) -> ()
        n191 = global write "质控中断报警全局.vi" "总磷总氮超时报警"(w243) -> ()
      }
    }
    n192 = Wait (ms)(milliseconds to wait=u32 1000 ("等待时间（毫秒）")) -> ()  [unwired: 1 out]
  }
  n193 = control-ref of="CODCr加标前水样浓度"() -> (w40:refnum<vi>)
  n194 = control-ref of="CODCr加标后水样浓度"() -> (w39:refnum<vi>)
  n195 = control-ref of="总氮加标水杯定容体积"() -> (w47:refnum<vi>)
  n196 = control-ref of="COD加标水杯定容体积"() -> (w63:refnum<vi>)
  n197 = control-ref of="总磷加标水杯定容体积"() -> (w72:refnum<vi>)
  n198 = control-ref of="氨氮加标水杯定容体积"() -> (w82:refnum<vi>)
  n199 = control-ref of="总氮加标前水样浓度"() -> (w49:refnum<vi>)
  n200 = control-ref of="总氮加标后水样浓度"() -> (w48:refnum<vi>)
  n201 = control-ref of="COD加标前水样浓度"() -> (w65:refnum<vi>)
  n202 = control-ref of="COD加标后水样浓度"() -> (w64:refnum<vi>)
  n203 = control-ref of="总磷加标前水样浓度"() -> (w74:refnum<vi>)
  n204 = control-ref of="总磷加标后水样浓度"() -> (w73:refnum<vi>)
  n205 = control-ref of="氨氮加标前水样浓度"() -> (w83:refnum<vi>)
  n206 = control-ref of="氨氮加标后水样浓度"() -> (w79:refnum<vi>)
  n207 = property on="窗格" class="Pane"("Origin"=T1 {"Horizontal"=0, "Vertical"=0} ("原点")) -> ()  [unwired: 2 in, 2 out]
  n208 = control-ref of="CODCr加标回收率"() -> (w35:refnum<vi>)
  n209 = control-ref of="CODCr母液浓度"() -> (w37:refnum<vi>)
  n210 = control-ref of="CODCr加标体积"() -> (w36:refnum<vi>)
  n211 = control-ref of="COD加标回收率"() -> (w60:refnum<vi>)
  n212 = control-ref of="总氮加标回收率"() -> (w44:refnum<vi>)
  n213 = control-ref of="总磷加标回收率"() -> (w70:refnum<vi>)
  n214 = control-ref of="氨氮加标回收率"() -> (w77:refnum<vi>)
  n215 = control-ref of="CODCr检出限"() -> (w41:refnum<vi>)
  n216 = control-ref of="总氮母液浓度"() -> (w46:refnum<vi>)
  n217 = control-ref of="总氮加标体积"() -> (w45:refnum<vi>)
  n218 = control-ref of="COD母液浓度"() -> (w62:refnum<vi>)
  n219 = control-ref of="COD加标体积"() -> (w61:refnum<vi>)
  n220 = control-ref of="总磷母液浓度"() -> (w71:refnum<vi>)
  n221 = control-ref of="总磷加标体积"() -> (w69:refnum<vi>)
  n222 = control-ref of="氨氮母液浓度"() -> (w81:refnum<vi>)
  n223 = control-ref of="氨氮加标体积"() -> (w78:refnum<vi>)
  n224 = control-ref of="CODCr量程"() -> (w42:refnum<vi>)
  n225 = control-ref of="总氮检出限"() -> (w50:refnum<vi>)
  n226 = control-ref of="COD检出限"() -> (w66:refnum<vi>)
  n227 = control-ref of="总磷检出限"() -> (w75:refnum<vi>)
  n228 = control-ref of="氨氮检出限"() -> (w84:refnum<vi>)
  n229 = control-ref of="总氮量程"() -> (w51:refnum<vi>)
  n230 = control-ref of="COD量程"() -> (w67:refnum<vi>)
  n231 = control-ref of="总磷量程"() -> (w76:refnum<vi>)
  n232 = control-ref of="氨氮量程"() -> (w85:refnum<vi>)
  n233 = property class="VI"(reference=w26) -> ("Name"=w27:string)  [unwired: 1 in, 2 out]
  n234 = Build Array(w42, w41, w40, w39, w38, w37, w36, w35) -> (w34:refnum<vi>[])
  n235 = Build Array(w51, w50, w49, w48, w47, w46, w45, w44) -> (w43:refnum<vi>[])
  n236 = Build Array(w67, w66, w65, w64, w63, w62, w61, w60) -> (w59:refnum<vi>[])
  n237 = Build Array(w76, w75, w74, w73, w72, w71, w69, w70) -> (w68:refnum<vi>[])
  n238 = Build Array(w85, w84, w83, w79, w82, w81, w78, w77) -> (w80:refnum<vi>[])
  n239 = property class="VI"(reference=w6) -> ("Name"=w7:string)  [unwired: 1 in, 2 out]
  n240 = Obtain Notifier(name (unnamed)="采配水Process" ("名称（未命名）"), notification data type=FALSE) -> (notifier out=w56:refnum<notifier>)  [unwired: 2 in, 2 out]
  n241 = Obtain Queue(name (unnamed)="质控单元" ("名称（未命名）"), element data type=cluster{"命令":string} {"命令"="启用模块"} ("元素")) -> (queue out=w23:refnum<queue>, error out=w22:errorcluster)  [unwired: 3 in, 1 out]
  n242 = Obtain Queue(name (unnamed)="采配水" ("名称（未命名）"), element data type=cluster{"命令":string, "数据":variant} {"命令"="", "数据"=variant}) -> (queue out=w53:refnum<queue>)  [unwired: 3 in, 2 out]
  n243 = control-ref of="CODCr加标后水样浓度"() -> (w5:refnum<vi>)
  n244 = property class="VI"(reference=w21) -> ("Name"=w20:string)  [unwired: 1 in, 2 out]
  n245 = control-ref of="总氮加标后水样浓度"() -> (w4:refnum<vi>)
  n246 = control-ref of="COD加标后水样浓度"() -> (w1:refnum<vi>)
  n247 = control-ref of="氨氮加标后水样浓度"() -> (w3:refnum<vi>)
  n248 = control-ref of="总磷加标后水样浓度"() -> (w2:refnum<vi>)
  n249 = Open VI Reference(type specifier VI Refnum (for type only)=refnum<vi> refnum, vi path=w27, options=128 ("选项")) -> (vi reference=w29:refnum<vi>, error out=w31:errorcluster)  [unwired: 3 in]
  n250 = Open VI Reference(type specifier VI Refnum (for type only)=refnum<vi> refnum, vi path=w7, options=128 ("选项")) -> (vi reference=w9:refnum<vi>, error out=w11:errorcluster)  [unwired: 3 in]
  n251 = while {
    tunnel: w23 -> [w313]
    tunnel: w22 -> [w312]
    stop <- FALSE stop-if-true
    # "通信入队列"
    n252 = Wait (ms)(milliseconds to wait=u32 1000 ("等待时间（毫秒）")) -> ()  [unwired: 1 out]
    n253 = local read "氨氮模块"() -> (w314:bool)
    n254 = case shown="真" w314 {
      tunnel: w313 -> [w345 w350]
      tunnel: w312 -> [w344 w349]
      tunnel: [w345 w348] -> w318
      tunnel: [w344 w347] -> w319
      frame False {
        w346 = FALSE ("通讯指示灯1")
        n255 = local write "氨氮传感器状态显示"(w346) -> ()
        n256 = local write "氨氮通讯"(w346) -> ()
      }
      frame True {
        n257 = Enqueue Element(queue=w350, element=cluster{"命令":string} {"命令"="氨氮读取"} ("元素"), error in (no error)=w349) -> (queue out=w348:refnum<queue>, error out=w347:errorcluster)  [unwired: 1 in, 1 out]
      }
    }
    n258 = local read "总磷总氮模块选择"() -> (w315:bool)
    n259 = case shown="假" w315 {
      tunnel: w318 -> [w337 w342]
      tunnel: w319 -> [w336 w341]
      tunnel: [w337 w340] -> w320
      tunnel: [w336 w339] -> w321
      frame False {
        w338 = FALSE ("通讯指示灯2")
        n260 = local write "总磷总氮通讯"(w338) -> ()
        n261 = local write "总磷总氮传感器状态显示"(w338) -> ()
      }
      frame True {
        n262 = Enqueue Element(queue=w342, element=cluster{"命令":string} {"命令"="总磷读取"} ("元素"), error in (no error)=w341) -> (queue out=w340:refnum<queue>, error out=w339:errorcluster)  [unwired: 1 in, 1 out]
      }
    }
    n263 = local read "CODMn选择"() -> (w316:bool)
    n264 = case shown="假" w316 {
      tunnel: w320 -> [w329 w334]
      tunnel: w321 -> [w328 w333]
      tunnel: [w329 w332] -> w322
      tunnel: [w328 w331] -> w323
      frame False {
        w330 = FALSE ("通讯指示灯3")
        n265 = local write "CODMn传感器状态显示"(w330) -> ()
        n266 = local write "CODMn通讯"(w330) -> ()
      }
      frame True {
        n267 = Enqueue Element(queue=w334, element=cluster{"命令":string} {"命令"="CODMn读取"} ("元素"), error in (no error)=w333) -> (queue out=w332:refnum<queue>, error out=w331:errorcluster)  [unwired: 1 in, 1 out]
      }
    }
    n268 = local read "CODCr选择"() -> (w317:bool)
    n269 = case shown="假" w317 {
      tunnel: w322 -> [_ w326]
      tunnel: w323 -> [_ w325]
      frame False {
        w324 = FALSE ("通讯指示灯3")
        n270 = local write "CODCr传感器状态显示"(w324) -> ()
        n271 = local write "CODCr通讯"(w324) -> ()
      }
      frame True {
        n272 = Enqueue Element(queue=w326, element=cluster{"命令":string} {"命令"="CODCr读取"} ("元素"), error in (no error)=w325) -> ()  [unwired: 1 in, 3 out]
      }
    }
  }
  n273 = while {
    tunnel: w80 -> [w360]
    tunnel: w68 -> [w359]
    tunnel: w59 -> [w354]
    tunnel: w56 -> [w358]
    tunnel: w53 -> [w357]
    tunnel: w43 -> [w356]
    tunnel: w34 -> [w355]
    tunnel: w23 -> [w353]
    tunnel: w22 -> [w352]
    stop <- FALSE stop-if-true
    # "氨氮站号是1，总磷总氮站号是2，CODMn站号是3，CODCr站号是4"
    n274 = event shown="[16] \"打开串口\": 值改变" {
      selector: _ -> [_ _ _ _ _ _ _ _ _ _ _ _ _ _ _ _ _ _ _ _ _ _ _ _]
      dyn-events: _ -> [_ _ _ _ _ _ _ _ _ _ _ _ _ _ _ _ _ _ _ _ _ _ _ _]
      timeout: _ -> [_ _ _ _ _ _ _ _ _ _ _ _ _ _ _ _ _ _ _ _ _ _ _ _]
      tunnel: w360 -> [_ _ _ _ _ _ _ _ _ _ w456 _ _ _ _ _ _ _ _ _ _ _ _ _]
      tunnel: w359 -> [_ _ _ _ _ _ _ _ _ _ _ w470 _ _ _ _ _ _ _ _ _ _ _ _]
      tunnel: w354 -> [_ _ _ _ _ _ _ _ _ _ _ _ _ w508 _ _ _ _ _ _ _ _ _ _]
      tunnel: w358 -> [_ _ _ _ _ _ _ _ _ _ _ _ _ _ _ _ _ _ w594 _ w685 w707 _ _]
      tunnel: w357 -> [_ _ _ _ _ _ _ _ _ _ _ _ _ _ _ _ _ _ _ _ _ w704 _ _]
      tunnel: w356 -> [_ _ _ _ _ _ _ _ _ _ _ _ w488 _ _ _ _ _ _ _ _ _ _ _]
      tunnel: [_ _ _ _ _ _ _ _ _ _ _ _ _ _ _ _ _ _ _ w619 _ _ _ _] -> _
      tunnel: w355 -> [_ _ _ _ _ _ _ _ _ _ _ _ _ _ w526 _ _ _ _ _ _ _ _ _]
      tunnel: w353 -> [_ _ _ _ _ _ _ _ _ _ _ _ _ _ _ _ w550 w584 _ _ _ _ _ _]
      tunnel: w352 -> [_ _ _ _ _ _ _ _ _ _ _ _ _ _ _ _ w549 w583 _ _ _ _ _ _]
      event Timeout {
        n275 = event-data() -> ()  [unwired: 1 in, 3 out]
      }
      event "氨氮量程", "氨氮检出限", "氨氮加标前水样浓度", "氨氮加标水杯定容体积", "氨氮母液浓度", "氨氮加标后水样浓度": Mouse Down {
        n276 = event-data() -> ("CtlRef"=w365:refnum<vi>)  [unwired: 1 in, 7 out]
        n277 = property class="DigNum (严格)"(reference=w365) -> (reference out=w363:refnum<vi>, "Value"=w364:dbl)  [unwired: 1 in, 1 out]
        n278 = call "数字键盘.vi"("OldNumber"=w364) -> ("NewNumber"=w362:sgl)
        n279 = property class="DigNum (严格)"(reference=w363, "Val(Sgnl)"=w362) -> ()  [unwired: 1 in, 2 out]
      }
      event "总磷母液浓度", "总磷加标水杯定容体积", "总磷加标后水样浓度", "总磷加标前水样浓度", "总磷检出限", "总磷量程": Mouse Down {
        n280 = event-data() -> ("CtlRef"=w369:refnum<vi>)  [unwired: 1 in, 7 out]
        n281 = property class="DigNum (严格)"(reference=w369) -> (reference out=w367:refnum<vi>, "Value"=w368:dbl)  [unwired: 1 in, 1 out]
        n282 = call "数字键盘.vi"("OldNumber"=w368) -> ("NewNumber"=w366:sgl)
        n283 = property class="DigNum (严格)"(reference=w367, "Val(Sgnl)"=w366) -> ()  [unwired: 1 in, 2 out]
      }
      event "总氮母液浓度", "总氮加标水杯定容体积", "总氮加标后水样浓度", "总氮加标前水样浓度", "总氮检出限", "总氮量程": Mouse Down {
        n284 = event-data() -> ("CtlRef"=w373:refnum<vi>)  [unwired: 1 in, 7 out]
        n285 = property class="DigNum (严格)"(reference=w373) -> (reference out=w371:refnum<vi>, "Value"=w372:dbl)  [unwired: 1 in, 1 out]
        n286 = call "数字键盘.vi"("OldNumber"=w372) -> ("NewNumber"=w370:sgl)
        n287 = property class="DigNum (严格)"(reference=w371, "Val(Sgnl)"=w370) -> ()  [unwired: 1 in, 2 out]
      }
      event "COD母液浓度", "COD加标水杯定容体积", "COD加标后水样浓度", "COD加标前水样浓度", "COD检出限", "COD量程": Mouse Down {
        n288 = event-data() -> ("CtlRef"=w377:refnum<vi>)  [unwired: 1 in, 7 out]
        n289 = property class="DigNum (严格)"(reference=w377) -> (reference out=w375:refnum<vi>, "Value"=w376:dbl)  [unwired: 1 in, 1 out]
        n290 = call "数字键盘.vi"("OldNumber"=w376) -> ("NewNumber"=w374:sgl)
        n291 = property class="DigNum (严格)"(reference=w375, "Val(Sgnl)"=w374) -> ()  [unwired: 1 in, 2 out]
      }
      event "CODCr检出限", "CODCr量程", "CODCr加标前水样浓度", "CODCr加标后水样浓度", "CODCr加标水杯定容体积", "CODCr母液浓度": Mouse Down {
        n292 = event-data() -> ("CtlRef"=w378:refnum<vi>)  [unwired: 1 in, 7 out]
        n293 = property class="DigNum (严格)"(reference=w378) -> (reference out=w380:refnum<vi>, "Value"=w381:dbl)  [unwired: 1 in, 1 out]
        n294 = call "数字键盘.vi"("OldNumber"=w381) -> ("NewNumber"=w379:sgl)
        n295 = property class="DigNum (严格)"(reference=w380, "Val(Sgnl)"=w379) -> ()  [unwired: 1 in, 2 out]
      }
      event "背隙补偿步数", "背隙补偿步数 2", "背隙补偿步数 3": Mouse Down {
        n296 = event-data() -> ("CtlRef"=w385:refnum<vi>)  [unwired: 1 in, 7 out]
        n297 = property class="DigNum (严格)"(reference=w385) -> (reference out=w384:refnum<vi>, "Value"=w383:i32)  [unwired: 1 in, 1 out]
        n298 = call "数字键盘.vi"("OldNumber"=w383) -> ("NewNumber"=w382:sgl)
        n299 = property class="DigNum (严格)"(reference=w384, "Val(Sgnl)"=w382) -> ()  [unwired: 1 in, 2 out]
      }
      event "背隙补偿步数", "背隙补偿步数 2", "背隙补偿步数 3": Value Change {
        w394 = "质控背隙补偿" ("section")
        n300 = event-data() -> ()  [unwired: 1 in, 6 out]
        n301 = call <vilib>:"Application Directory.vi"() -> ("Application Directory"=w401:path)
        n302 = Build Path(base path=w401, name or relative path="data\\Set.ini" ("名称或相对路径")) -> (appended path=w399:path)
        n303 = call <vilib>:"Open Config Data.vi"("configuration file path"=w399) -> ("error out"=w397:errorcluster, "refnum"=w398:T2)  [unwired: 8 in, 1 out]
        n304 = call-poly <vilib>:"Write Key.vi"("section"=w394, "error in (no error)"=w397, "value"="背隙补偿步数", "key"="背隙值1", "refnum"=w398) -> ("error out"=w388:errorcluster, "refnum out"=w391:T2)  [unwired: 4 in, 1 out]
        n305 = call-poly <vilib>:"Write Key.vi"("section"=w394, "error in (no error)"=w388, "value"="背隙补偿步数 2", "key"="背隙值2", "refnum"=w391) -> ("error out"=w389:errorcluster, "refnum out"=w390:T2)  [unwired: 4 in, 1 out]
        n306 = call-poly <vilib>:"Write Key.vi"("section"=w394, "error in (no error)"=w389, "value"="背隙补偿步数 3", "key"="背隙值3", "refnum"=w390) -> ()  [unwired: 4 in, 3 out]
      }
      event "氨氮模块", "总磷总氮模块选择", "CODMn选择", "CODCr选择": Value Change {
        w405 = "质控模块选择" ("section")
        n307 = event-data() -> ()  [unwired: 1 in, 6 out]
        n308 = call <vilib>:"Application Directory.vi"() -> ("Application Directory"=w423:path)
        n309 = Build Path(base path=w423, name or relative path="data\\Set.ini" ("名称或相对路径")) -> (appended path=w421:path)
        n310 = local read "氨氮模块"() -> (w411:bool)
        n311 = call <vilib>:"Open Config Data.vi"("configuration file path"=w421) -> ("error out"=w419:errorcluster, "refnum"=w420:T2)  [unwired: 8 in, 1 out]
        n312 = local read "总磷总氮模块选择"() -> (w410:bool)
        n313 = call-poly <vilib>:"Write Key.vi"("section"=w405, "error in (no error)"=w419, "value"=w411, "key"="模块1" ("section"), "refnum"=w420) -> ("error out"=w417:errorcluster, "refnum out"=w418:T2)  [unwired: 4 in, 1 out]
        n314 = local read "CODMn选择"() -> (w409:bool)
        n315 = call-poly <vilib>:"Write Key.vi"("section"=w405, "error in (no error)"=w417, "value"=w410, "key"="模块2" ("section"), "refnum"=w418) -> ("error out"=w415:errorcluster, "refnum out"=w416:T2)  [unwired: 4 in, 1 out]
        n316 = local read "CODCr选择"() -> (w402:bool)
        n317 = call-poly <vilib>:"Write Key.vi"("section"=w405, "error in (no error)"=w415, "value"=w409, "key"="模块3" ("section"), "refnum"=w416) -> ("error out"=w406:errorcluster, "refnum out"=w407:T2)  [unwired: 4 in, 1 out]
        n318 = call-poly <vilib>:"Write Key.vi"("section"=w405, "error in (no error)"=w406, "value"=w402, "key"="模块4" ("section"), "refnum"=w407) -> ("error out"=w403:errorcluster, "refnum out"=w404:T2)  [unwired: 4 in, 1 out]
        n319 = call <vilib>:"Close Config Data.vi"("error in (no error)"=w403, "refnum"=w404) -> ()  [unwired: 8 in, 2 out]
      }
      event "氨氮量程选择", "总氮量程选择", "总磷量程选择", "CODMn量程选择", "CODCr量程选择": Value Change {
        w430 = "质控模块量程选择" ("section")
        n320 = event-data() -> ()  [unwired: 1 in, 6 out]
        n321 = call <vilib>:"Application Directory.vi"() -> ("Application Directory"=w449:path)
        n322 = Build Path(base path=w449, name or relative path="data\\Set.ini" ("名称或相对路径")) -> (appended path=w447:path)
        n323 = local read "氨氮量程选择"() -> (w434:enum32{"H", "L", "AUTO"})
        n324 = call <vilib>:"Open Config Data.vi"("configuration file path"=w447) -> ("error out"=w445:errorcluster, "refnum"=w446:T2)  [unwired: 8 in, 1 out]
        n325 = local read "总氮量程选择"() -> (w433:enum32{"H", "L", "AUTO"})
        n326 = call-poly <vilib>:"Write Key.vi"("section"=w430, "error in (no error)"=w445, "value"=w434, "key"="氨氮" ("section"), "refnum"=w446) -> ("error out"=w443:errorcluster, "refnum out"=w444:T2)  [unwired: 4 in, 1 out]
        n327 = local read "总磷量程选择"() -> (w432:enum32{"H", "L", "AUTO"})
        n328 = call-poly <vilib>:"Write Key.vi"("section"=w430, "error in (no error)"=w443, "value"=w433, "key"="总氮" ("section"), "refnum"=w444) -> ("error out"=w441:errorcluster, "refnum out"=w442:T2)  [unwired: 4 in, 1 out]
        n329 = local read "CODMn量程选择"() -> (w431:enum32{"H", "L", "AUTO"})
        n330 = call-poly <vilib>:"Write Key.vi"("section"=w430, "error in (no error)"=w441, "value"=w432, "key"="总磷" ("section"), "refnum"=w442) -> ("error out"=w436:errorcluster, "refnum out"=w437:T2)  [unwired: 4 in, 1 out]
        n331 = local read "CODCr量程选择"() -> (w424:enum32{"H", "L", "AUTO"})
        n332 = call-poly <vilib>:"Write Key.vi"("section"=w430, "error in (no error)"=w436, "value"=w431, "key"="CODMn" ("section"), "refnum"=w437) -> ("error out"=w426:errorcluster, "refnum out"=w429:T2)  [unwired: 4 in, 1 out]
        n333 = call-poly <vilib>:"Write Key.vi"("section"=w430, "error in (no error)"=w426, "value"=w424, "key"="CODCr" ("section"), "refnum"=w429) -> ("error out"=w427:errorcluster, "refnum out"=w428:T2)  [unwired: 4 in, 1 out]
        n334 = call <vilib>:"Close Config Data.vi"("error in (no error)"=w427, "refnum"=w428) -> ()  [unwired: 8 in, 2 out]
      }
      event "氨氮量程", "氨氮检出限", "氨氮加标前水样浓度", "氨氮母液浓度", "氨氮加标水杯定容体积", "氨氮加标后水样浓度": Value Change {
        n335 = event-data() -> ()  [unwired: 1 in, 6 out]
        n336 = for {
          tunnel: w456 -> [w468] mode=indexing
          tunnel: [w467] -> w465 mode=indexing
          n337 = property class="DigNum (严格)"(reference=w468) -> ("Value"=w467:dbl)  [unwired: 1 in, 2 out]
        }
        n338 = Index Array(array=w465) -> (element #1=w464:dbl, element #2=w463:dbl, element #3=w450:dbl, element #4=w462:dbl, element #5=w461:dbl, element #6=w459:dbl)  [unwired: 6 in]
        n339 = global write "水样浓度全局.vi" "氨氮加标前水样浓度"(w450) -> ()
        n340 = Bundle By Name(cluster=T3 {"量程"=0.0, "检出限"=0.0, "加标前水样浓度"=0.0, "加标后水样浓度"=0.0, "加标水杯定容体积"=0.0, "加标母液浓度"=0.0, "加标体积"=0.0, "加标回收率"=0.0} ("参数"), "量程"=w464, "检出限"=w463, "加标前水样浓度"=w450, "加标后水样浓度"=w462, "加标水杯定容体积"=w461, "加标母液浓度"=w459) -> (w458:T3)
        n341 = call "加标回收率计算.vi"("参数"=w458) -> ("参数 out"=w457:T3)  [unwired: 10 in]
        n342 = call "质控参数保存.vi"("section"="氨氮质控参数", "参数"=w457) -> ()  [unwired: 9 in, 1 out]
        n343 = Unbundle By Name(w457) -> ("加标体积"=w451:dbl, "加标回收率"=w452:dbl)
        n344 = Index Array(array=w456, index #1=6 ("索引")) -> (element #1=w455:refnum<vi>, element #2=w453:refnum<vi>)  [unwired: 1 in]
        n345 = property class="DigNum (严格)"(reference=w455, "Value"=w451) -> ()  [unwired: 1 in, 2 out]
        n346 = property class="DigNum (严格)"(reference=w453, "Value"=w452) -> ()  [unwired: 1 in, 2 out]
      }
      event "总磷母液浓度", "总磷加标水杯定容体积", "总磷加标后水样浓度", "总磷加标前水样浓度", "总磷检出限", "总磷量程": Value Change {
        n347 = event-data() -> ()  [unwired: 1 in, 6 out]
        n348 = for {
          tunnel: w470 -> [w487] mode=indexing
          tunnel: [w486] -> w484 mode=indexing
          n349 = property class="DigNum (严格)"(reference=w487) -> ("Value"=w486:dbl)  [unwired: 1 in, 2 out]
        }
        n350 = Index Array(array=w484) -> (element #1=w483:dbl, element #2=w482:dbl, element #3=w469:dbl, element #4=w481:dbl, element #5=w480:dbl, element #6=w478:dbl)  [unwired: 6 in]
        n351 = global write "水样浓度全局.vi" "总磷加标前水样浓度"(w469) -> ()
        n352 = Bundle By Name(cluster=T3 {"量程"=0.0, "检出限"=0.0, "加标前水样浓度"=0.0, "加标后水样浓度"=0.0, "加标水杯定容体积"=0.0, "加标母液浓度"=0.0, "加标体积"=0.0, "加标回收率"=0.0} ("参数"), "量程"=w483, "检出限"=w482, "加标前水样浓度"=w469, "加标后水样浓度"=w481, "加标水杯定容体积"=w480, "加标母液浓度"=w478) -> (w477:T3)
        n353 = call "加标回收率计算.vi"("参数"=w477) -> ("参数 out"=w476:T3)  [unwired: 10 in]
        n354 = call "质控参数保存.vi"("section"="总磷质控参数", "参数"=w476) -> ()  [unwired: 9 in, 1 out]
        n355 = Unbundle By Name(w476) -> ("加标体积"=w473:dbl, "加标回收率"=w471:dbl)
        n356 = Index Array(array=w470, index #1=6 ("索引")) -> (element #1=w475:refnum<vi>, element #2=w472:refnum<vi>)  [unwired: 1 in]
        n357 = property class="DigNum (严格)"(reference=w475, "Value"=w473) -> ()  [unwired: 1 in, 2 out]
        n358 = property class="DigNum (严格)"(reference=w472, "Value"=w471) -> ()  [unwired: 1 in, 2 out]
      }
      event "总氮量程", "总氮检出限", "总氮加标前水样浓度", "总氮加标后水样浓度", "总氮加标水杯定容体积", "总氮母液浓度": Value Change {
        n359 = event-data() -> ()  [unwired: 1 in, 6 out]
        n360 = for {
          tunnel: w488 -> [w506] mode=indexing
          tunnel: [w505] -> w503 mode=indexing
          n361 = property class="DigNum (严格)"(reference=w506) -> ("Value"=w505:dbl)  [unwired: 1 in, 2 out]
        }
        n362 = Index Array(array=w503) -> (element #1=w502:dbl, element #2=w501:dbl, element #3=w489:dbl, element #4=w500:dbl, element #5=w499:dbl, element #6=w497:dbl)  [unwired: 6 in]
        n363 = global write "水样浓度全局.vi" "总氮加标前水样浓度"(w489) -> ()
        n364 = Bundle By Name(cluster=T3 {"量程"=0.0, "检出限"=0.0, "加标前水样浓度"=0.0, "加标后水样浓度"=0.0, "加标水杯定容体积"=0.0, "加标母液浓度"=0.0, "加标体积"=0.0, "加标回收率"=0.0} ("参数"), "量程"=w502, "检出限"=w501, "加标前水样浓度"=w489, "加标后水样浓度"=w500, "加标水杯定容体积"=w499, "加标母液浓度"=w497) -> (w496:T3)
        n365 = call "加标回收率计算.vi"("参数"=w496) -> ("参数 out"=w495:T3)  [unwired: 10 in]
        n366 = call "质控参数保存.vi"("section"="总氮质控参数", "参数"=w495) -> ()  [unwired: 9 in, 1 out]
        n367 = Unbundle By Name(w495) -> ("加标体积"=w492:dbl, "加标回收率"=w490:dbl)
        n368 = Index Array(array=w488, index #1=6 ("索引")) -> (element #1=w494:refnum<vi>, element #2=w491:refnum<vi>)  [unwired: 1 in]
        n369 = property class="DigNum (严格)"(reference=w494, "Value"=w492) -> ()  [unwired: 1 in, 2 out]
        n370 = property class="DigNum (严格)"(reference=w491, "Value"=w490) -> ()  [unwired: 1 in, 2 out]
      }
      event "COD母液浓度", "COD加标水杯定容体积", "COD加标后水样浓度", "COD加标前水样浓度", "COD检出限", "COD量程": Value Change {
        n371 = event-data() -> ()  [unwired: 1 in, 6 out]
        n372 = for {
          tunnel: w508 -> [w525] mode=indexing
          tunnel: [w524] -> w522 mode=indexing
          n373 = property class="DigNum (严格)"(reference=w525) -> ("Value"=w524:dbl)  [unwired: 1 in, 2 out]
        }
        n374 = Index Array(array=w522) -> (element #1=w521:dbl, element #2=w520:dbl, element #3=w507:dbl, element #4=w519:dbl, element #5=w518:dbl, element #6=w516:dbl)  [unwired: 6 in]
        n375 = global write "水样浓度全局.vi" "COD加标前水样浓度"(w507) -> ()
        n376 = Bundle By Name(cluster=T3 {"量程"=0.0, "检出限"=0.0, "加标前水样浓度"=0.0, "加标后水样浓度"=0.0, "加标水杯定容体积"=0.0, "加标母液浓度"=0.0, "加标体积"=0.0, "加标回收率"=0.0} ("参数"), "量程"=w521, "检出限"=w520, "加标前水样浓度"=w507, "加标后水样浓度"=w519, "加标水杯定容体积"=w518, "加标母液浓度"=w516) -> (w515:T3)
        n377 = call "加标回收率计算.vi"("参数"=w515) -> ("参数 out"=w514:T3)  [unwired: 10 in]
        n378 = call "质控参数保存.vi"("section"="COD质控参数", "参数"=w514) -> ()  [unwired: 9 in, 1 out]
        n379 = Unbundle By Name(w514) -> ("加标体积"=w511:dbl, "加标回收率"=w509:dbl)
        n380 = Index Array(array=w508, index #1=6 ("索引")) -> (element #1=w513:refnum<vi>, element #2=w510:refnum<vi>)  [unwired: 1 in]
        n381 = property class="DigNum (严格)"(reference=w513, "Value"=w511) -> ()  [unwired: 1 in, 2 out]
        n382 = property class="DigNum (严格)"(reference=w510, "Value"=w509) -> ()  [unwired: 1 in, 2 out]
      }
      event "CODCr母液浓度", "CODCr加标水杯定容体积", "CODCr加标前水样浓度", "CODCr检出限", "CODCr量程", "CODCr加标后水样浓度": Value Change {
        n383 = event-data() -> ()  [unwired: 1 in, 6 out]
        n384 = for {
          tunnel: w526 -> [w544] mode=indexing
          tunnel: [w543] -> w541 mode=indexing
          n385 = property class="DigNum (严格)"(reference=w544) -> ("Value"=w543:dbl)  [unwired: 1 in, 2 out]
        }
        n386 = Index Array(array=w541) -> (element #1=w540:dbl, element #2=w539:dbl, element #3=w527:dbl, element #4=w538:dbl, element #5=w537:dbl, element #6=w535:dbl)  [unwired: 6 in]
        n387 = global write "水样浓度全局.vi" "CODCr加标前水样浓度"(w527) -> ()
        n388 = Bundle By Name(cluster=T3 {"量程"=0.0, "检出限"=0.0, "加标前水样浓度"=0.0, "加标后水样浓度"=0.0, "加标水杯定容体积"=0.0, "加标母液浓度"=0.0, "加标体积"=0.0, "加标回收率"=0.0} ("参数"), "量程"=w540, "检出限"=w539, "加标前水样浓度"=w527, "加标后水样浓度"=w538, "加标水杯定容体积"=w537, "加标母液浓度"=w535) -> (w534:T3)
        n389 = call "加标回收率计算.vi"("参数"=w534) -> ("参数 out"=w533:T3)  [unwired: 10 in]
        n390 = call "质控参数保存.vi"("section"="CODCr质控参数", "参数"=w533) -> ()  [unwired: 9 in, 1 out]
        n391 = Unbundle By Name(w533) -> ("加标体积"=w530:dbl, "加标回收率"=w528:dbl)
        n392 = Index Array(array=w526, index #1=6 ("索引")) -> (element #1=w532:refnum<vi>, element #2=w529:refnum<vi>)  [unwired: 1 in]
        n393 = property class="DigNum (严格)"(reference=w532, "Value"=w530) -> ()  [unwired: 1 in, 2 out]
        n394 = property class="DigNum (严格)"(reference=w529, "Value"=w528) -> ()  [unwired: 1 in, 2 out]
      }
      event "手动调试": Value Change {
        n395 = event-data() -> ()  [unwired: 1 in, 6 out]
        n396 = call "手动调试界面.vi"() -> ()  [unwired: 16 in]
      }
      event "打开串口": Value Change {
        n397 = event-data() -> ()  [unwired: 1 in, 6 out]
        n398 = global read "断电保存全局.vi" "MB通信方式选择"() -> (w545:enum16{"串口", "TCP"})
        n399 = global read "断电保存全局.vi" "VISA Resource"() -> (w546:refnum<visa-resource-name>)
        n400 = global read "断电保存全局.vi" "PORT"() -> (w547:string)
        n401 = global read "断电保存全局.vi" "IP"() -> (w548:string)
        n402 = call "串口配置.vi"("PORT"=w547, "IP"=w548, "MB通信方式选择"=w545, "请选择串口:"=w546) -> ("PORT 2"=w552:string, "IP 2"=w553:string, "确认 2"=w555:bool, "VISA资源名称 2"=w554:refnum<visa-resource-name>, "MB通信方式选择 2"=w551:enum16{"串口", "TCP"})  [unwired: 3 in]
        n403 = case shown="真" w555 {
          tunnel: w554 -> [_ w561]
          tunnel: w550 -> [_ w560]
          tunnel: w553 -> [_ w559]
          tunnel: w552 -> [_ w558]
          tunnel: w551 -> [_ w557]
          tunnel: w549 -> [_ w556]
          frame False {
          }
          frame True {
            n404 = flat-sequence {
              tunnel: w561 -> [w565]
              tunnel: w560 -> [w567]
              tunnel: w559 -> [w564]
              tunnel: w558 -> [w563]
              tunnel: w557 -> [w562]
              tunnel: w556 -> [w566]
              frame #0 {
                n405 = global write "断电保存全局.vi" "IP"(w564) -> ()
                n406 = global write "断电保存全局.vi" "PORT"(w563) -> ()
                n407 = global write "断电保存全局.vi" "VISA Resource"(w565) -> ()
                n408 = global write "断电保存全局.vi" "MB通信方式选择"(w562) -> ()
                n409 = Enqueue Element(queue=w567, element=cluster{"命令":string} {"命令"="启用模块"} ("元素"), error in (no error)=w566) -> ()  [unwired: 1 in, 3 out]
              }
              frame #1 {
                n410 = call <vilib>:"Application Directory.vi"() -> ("Application Directory"=w582:path)
                n411 = Build Path(base path=w582, name or relative path="data\\sys.ini" ("名称或相对路径")) -> (appended path=w580:path)
                n412 = call <vilib>:"Open Config Data.vi"("configuration file path"=w580) -> ("error out"=w576:errorcluster, "refnum"=w579:T2)  [unwired: 8 in, 1 out]
                n413 = vi-ref "质控单元.lvlib:断电保存全局.vi"() -> (w578:refnum<vi>)
                n414 = call <userlib>:"Write Panel to INI__ogtk.vi"("error in (no error)"=w576, "VI ref"=w578, "refnum"=w579) -> ("error out"=w575:errorcluster, "refnum out"=w577:T2)  [unwired: 7 in]
                n415 = call <vilib>:"Close Config Data.vi"("error in (no error)"=w575, "refnum"=w577) -> ("error out"=w570:errorcluster, "file path"=w569:path)  [unwired: 8 in]
                n416 = Open/Create/Replace File(file path (use dialog)=w569, error in=w570) -> (refnum out=w573:refnum<file>, error out=w574:errorcluster)  [unwired: 4 in, 1 out]
                n417 = Flush File(refnum=w573, error in=w574) -> (refnum out=w572:refnum<file>, error out=w571:errorcluster)
                n418 = Close File(refnum=w572, error in=w571) -> ()  [unwired: 2 out]
              }
            }
          }
        }
      }
      event "释放串口": Value Change {
        n419 = event-data() -> ()  [unwired: 1 in, 6 out]
        n420 = Two Button Dialog(message="确认是否释放串口，释放串口将导致通信失败！" ("消息")) -> (T button?=w585:bool)  [unwired: 2 in]
        n421 = case shown="真" w585 {
          tunnel: w584 -> [_ w588]
          tunnel: w583 -> [_ w587]
          frame False {
          }
          frame True {
            n422 = Bundle By Name(cluster=cluster{"命令":string} {"命令"=""} ("元素"), "命令"="停用模块" ("名称（未命名）")) -> (w589:cluster{"命令":string})
            n423 = Enqueue Element(queue=w588, element=w589, error in (no error)=w587) -> ()  [unwired: 1 in, 3 out]
          }
        }
      }
      event "加标回收": Value Change {
        n424 = event-data() -> ()  [unwired: 1 in, 6 out]
        n425 = Send Notification(notification=FALSE ("通知"), notifier=w594) -> ()  [unwired: 1 in, 2 out]
        n426 = call "质控启动流程对话框.vi"() -> ("确定启动"=w592:bool, "启动模块"=w597:T8, "直接启动"=w595:bool, "常规启动"=w596:bool)  [unwired: 8 in]
        n427 = case shown="真" w592 {
          tunnel: w597 -> [_ w606]
          tunnel: w596 -> [_ w605]
          tunnel: w595 -> [_ w604]
          frame False {
          }
          frame True {
            n428 = Bundle By Name(cluster=T5 {"是否启用仪器"=FALSE, "CODMn"={"启动测量模式"={"测量模式"=enum."水样测量"}, "确定按钮"=FALSE}, "启动模块"={"氨氮"=FALSE, "总磷"=FALSE, "总氮"=FALSE, "CODMn"=FALSE, "CODCr"=FALSE}, "常规启动"=FALSE, "直接启动"=FALSE} ("参数"), "是否启用仪器"=TRUE, "启动模块"=w606, "常规启动"=w605, "直接启动"=w604) -> (w598:T5)
            n429 = vi-ref "质控单元.lvlib:一体站流程质控自动启动.vi"() -> (w601:refnum<vi>)
            n430 = property class="VI"(reference=w601) -> ("Name"=w602:string, "Exec.State"=w600:T9)  [unwired: 1 in, 2 out]
            n431 = case shown="\"Idle\"" w600 {
              tunnel: w602 -> [_ w617]
              tunnel: w598 -> [_ w607]
              frame "Bad", Default {
              }
              frame "Idle" {
                n432 = Open VI Reference(type specifier VI Refnum (for type only)=refnum<vi> refnum ("类型说明符VI引用句柄（仅用于类型）"), vi path=w617, options=128 ("选项")) -> (vi reference=w618:refnum<vi>, error out=w614:errorcluster)  [unwired: 3 in]
                n433 = call-by-ref "开始异步调用"(reference=w618, error in=w614, "CODMn量程切换"="CODMn量程选择", "总磷量程切换"="总磷量程选择", "总氮量程切换"="总氮量程选择", "氨氮量程切换"="氨氮量程选择", "参数"=w607) -> (reference out=w616:refnum<vi>, error out=w615:errorcluster)  [unwired: 7 in]
                n434 = Close Reference(reference=w616, error in (no error)=w615) -> ()  [unwired: 1 out]
              }
            }
          }
        }
      }
      event "报警清除": Value Change {
        w625 = FALSE ("氨氮中断报警")
        n435 = event-data() -> ()  [unwired: 1 in, 6 out]
        n436 = global write "质控中断报警全局.vi" "氨氮中断报警"(w625) -> ()
        n437 = global write "质控中断报警全局.vi" "CODMn中断报警"(w625) -> ()
        n438 = global write "质控中断报警全局.vi" "总氮中断报警"(w625) -> ()
        n439 = global write "质控中断报警全局.vi" "总磷中断报警"(w625) -> ()
        n440 = global write "质控中断报警全局.vi" "CODCr中断报警"(w625) -> ()
        n441 = local read "氨氮模块"() -> (w635:bool)
        n442 = case shown="真" w635 {
          tunnel: [errorcluster {"status"=FALSE, "code"=0, "source"=""} ("error out") w678] -> w632
          frame False {
          }
          frame True {
            n443 = call "多个线圈写入.vi"("values"=bool[] [TRUE], "starting address"=u16 2106, "Slave ID"=u8 1) -> ("error out"=w678:errorcluster)  [unwired: 8 in]
          }
        }
        n444 = local read "总磷总氮模块选择"() -> (w634:bool)
        n445 = case shown="真" w634 {
          tunnel: w632 -> [w671 w674]
          tunnel: [w671 w672] -> w631
          frame False {
          }
          frame True {
            n446 = call "多个线圈写入.vi"("Error in"=w674, "values"=bool[] [TRUE], "starting address"=u16 2106, "Slave ID"=u8 2) -> ("error out"=w672:errorcluster)  [unwired: 7 in]
          }
        }
        n447 = local read "CODMn选择"() -> (w633:bool)
        n448 = case shown="真" w633 {
          tunnel: w631 -> [w665 w669]
          tunnel: [w665 w666] -> w622
          frame False {
          }
          frame True {
            n449 = call "多个线圈写入.vi"("Error in"=w669, "values"=bool[] [TRUE], "starting address"=u16 2106, "Slave ID"=u8 3) -> ("error out"=w666:errorcluster)  [unwired: 7 in]
          }
        }
        n450 = local read "CODCr选择"() -> (w623:bool)
        n451 = case shown="真" w623 {
          tunnel: w622 -> [w642 w646]
          tunnel: [w642 w643] -> w621
          frame False {
          }
          frame True {
            n452 = call "多个线圈写入.vi"("Error in"=w646, "values"=bool[] [TRUE], "starting address"=u16 2106, "Slave ID"=u8 4) -> ("error out"=w643:errorcluster)  [unwired: 7 in]
          }
        }
        n453 = local read "氨氮模块"() -> (w626:bool)
        n454 = case shown="真" w626 {
          tunnel: [w660 w661] -> w629
          tunnel: w621 -> [w660 _]
          frame False {
          }
          frame True {
            n455 = call "多个线圈写入.vi"("values"=bool[] [FALSE], "starting address"=u16 2106, "Slave ID"=u8 1) -> ("error out"=w661:errorcluster)  [unwired: 8 in]
          }
        }
        n456 = local read "总磷总氮模块选择"() -> (w627:bool)
        n457 = case shown="真" w627 {
          tunnel: w629 -> [w654 w657]
          tunnel: [w654 w655] -> w630
          frame False {
          }
          frame True {
            n458 = call "多个线圈写入.vi"("Error in"=w657, "values"=bool[] [FALSE], "starting address"=u16 2106, "Slave ID"=u8 2) -> ("error out"=w655:errorcluster)  [unwired: 7 in]
          }
        }
        n459 = local read "CODMn选择"() -> (w628:bool)
        n460 = case shown="真" w628 {
          tunnel: w630 -> [w648 w652]
          tunnel: [w648 w649] -> w620
          frame False {
          }
          frame True {
            n461 = call "多个线圈写入.vi"("Error in"=w652, "values"=bool[] [FALSE], "starting address"=u16 2106, "Slave ID"=u8 3) -> ("error out"=w649:errorcluster)  [unwired: 7 in]
          }
        }
        n462 = local read "CODCr选择"() -> (w624:bool)
        n463 = case shown="真" w624 {
          tunnel: w620 -> [w636 w640]
          tunnel: [w636 w637] -> w619
          frame False {
          }
          frame True {
            n464 = call "多个线圈写入.vi"("Error in"=w640, "values"=bool[] [FALSE], "starting address"=u16 2106, "Slave ID"=u8 4) -> ("error out"=w637:errorcluster)  [unwired: 7 in]
          }
        }
      }
      event "平行样测试": Value Change {
        n465 = event-data() -> ()  [unwired: 1 in, 6 out]
        n466 = Cancel Notification(0:w685) -> ()  [unwired: 1 in, 3 out]
        n467 = call "平行样启动流程对话框.vi"() -> ("启动模块"=w684:T10, "常规启动"=w682:bool, "确定启动"=w683:bool)  [unwired: 9 in]
        n468 = case shown="真" w683 {
          tunnel: w684 -> [_ w687]
          tunnel: w682 -> [_ w686]
          frame False {
          }
          frame True {
            (unwired) TRUE ("是否启用仪器")
            n469 = Bundle By Name(cluster=T6 {"参数启用"={"CODMn"=FALSE, "总磷"=FALSE, "总氮"=FALSE, "氨氮"=FALSE, "CODcr"=FALSE}, "采配水是否启动"=FALSE} ("参数"), "参数启用"=w687, "采配水是否启动"=w686) -> (w690:T6)
            n470 = vi-ref "一体站流程平行样自动启动.vi"() -> (w691:refnum<vi>)
            n471 = property class="VI"(reference=w691) -> ("Name"=w692:string, "Exec.State"=w689:T9)  [unwired: 1 in, 2 out]
            n472 = case shown="\"Idle\"" w689 {
              tunnel: w692 -> [_ w699]
              tunnel: w690 -> [_ w693]
              frame "Bad", Default {
              }
              frame "Idle" {
                n473 = Open VI Reference(type specifier VI Refnum (for type only)=refnum<vi> refnum ("类型说明符VI引用句柄（仅用于类型）"), vi path=w699, options=128 ("选项")) -> (vi reference=w700:refnum<vi>, error out=w698:errorcluster)  [unwired: 3 in]
                n474 = call-by-ref "开始异步调用"(reference=w700, error in=w698, "参数"=w693) -> (reference out=w695:refnum<vi>, error out=w694:errorcluster)  [unwired: 11 in]
                n475 = Close Reference(reference=w695, error in (no error)=w694) -> ()  [unwired: 1 out]
              }
            }
          }
        }
      }
      event "停止测量": Value Change {
        w701 = TRUE ("氨氮")
        # "停止采配水、氨氮、总磷总氮、COD、质控"
        n476 = event-data() -> ()  [unwired: 1 in, 6 out]
        n477 = Send Notification(notification=TRUE ("通知"), notifier=w707) -> ()  [unwired: 1 in, 2 out]
        n478 = call "质控启动参数选择对话框.vi"("CODCr"=w701, "CODMn"=w701, "总氮"=w701, "总磷"=w701, "氨氮"=w701) -> ("确定启动"=w702:bool, "启动模块"=w703:T8)  [unwired: 4 in, 1 out]
        n479 = case shown="真" w702 {
          tunnel: w703 -> [_ w714]
          frame False {
          }
          frame True {
            n480 = Unbundle By Name(w714) -> ("氨氮"=w712:bool, "总磷"=w711:bool, "总氮"=w710:bool, "CODMn"=w713:bool, "CODCr"=w708:bool)
            n481 = case shown="真" w713 {
              frame False {
              }
              frame True {
                n482 = call "CODMn停止命令 (子VI).vi"() -> ()  [unwired: 12 in]
                n483 = call "单个写入.vi"("value"=u16 2, "address"=u16 103, "Slave ID"=u8 3) -> ()  [unwired: 8 in, 1 out]
                n484 = Obtain Notifier(name (unnamed)="CODMn" ("名称（未命名）"), notification data type=FALSE) -> (notifier out=w747:refnum<notifier>)  [unwired: 2 in, 2 out]
                n485 = Send Notification(notification=TRUE ("通知"), notifier=w747) -> ()  [unwired: 1 in, 2 out]
              }
            }
            n486 = case shown="真" w708 {
              frame False {
              }
              frame True {
                n487 = call "CODCr停止命令 (子VI).vi"() -> ()  [unwired: 12 in]
                n488 = call "单个写入.vi"("value"=u16 2, "address"=u16 103, "Slave ID"=u8 4) -> ()  [unwired: 8 in, 1 out]
                n489 = Obtain Notifier(name (unnamed)="CODCr" ("名称（未命名）"), notification data type=FALSE) -> (notifier out=w718:refnum<notifier>)  [unwired: 2 in, 2 out]
                n490 = Send Notification(notification=TRUE ("通知"), notifier=w718) -> ()  [unwired: 1 in, 2 out]
              }
            }
            n491 = case shown="真" w712 {
              frame False {
              }
              frame True {
                n492 = call "单个写入.vi"("value"=u16 2, "address"=u16 103, "Slave ID"=u8 1) -> ()  [unwired: 8 in, 1 out]
                n493 = Obtain Queue(name (unnamed)="NH3N" ("名称（未命名）"), element data type=cluster{"命令":string, "data":variant} {"命令"="", "data"=variant}) -> (queue out=w743:refnum<queue>)  [unwired: 3 in, 2 out]
                n494 = Obtain Notifier(name (unnamed)="NH3N" ("名称（未命名）"), notification data type=FALSE) -> (notifier out=w739:refnum<notifier>)  [unwired: 2 in, 2 out]
                n495 = Send Notification(notification=TRUE ("通知"), notifier=w739) -> ()  [unwired: 1 in, 2 out]
                n496 = Enqueue Element(queue=w743, element=cluster{"命令":string, "data":variant} {"命令"="启动", "data"=variant(cluster{"站号":u16, "控制命令输出":u16[]} {"站号"=1, "控制命令输出"=[2816]})} ("元素")) -> ()  [unwired: 2 in, 3 out]
              }
            }
            n497 = Or(x=w711, y=w710) -> (x .or. y?=w709:bool)
            n498 = case shown="真" w709 {
              frame False {
              }
              frame True {
                n499 = call "单个写入.vi"("value"=u16 2, "address"=u16 103, "Slave ID"=u8 2) -> ()  [unwired: 8 in, 1 out]
                n500 = Obtain Queue(name (unnamed)="TP" ("名称（未命名）"), element data type=cluster{"命令":string, "data":variant} {"命令"="", "data"=variant}) -> (queue out=w732:refnum<queue>)  [unwired: 3 in, 2 out]
                n501 = Obtain Notifier(name (unnamed)="TNTP" ("名称（未命名）"), notification data type=FALSE) -> (notifier out=w728:refnum<notifier>)  [unwired: 2 in, 2 out]
                n502 = Send Notification(notification=TRUE ("通知"), notifier=w728) -> ()  [unwired: 1 in, 2 out]
                n503 = Enqueue Element(queue=w732, element=cluster{"命令":string, "data":variant} {"命令"="启动", "data"=variant(cluster{"站号":u16, "控制命令输出":u16[]} {"站号"=1, "控制命令输出"=[2816]})} ("元素")) -> ()  [unwired: 2 in, 3 out]
              }
            }
          }
        }
        n504 = Enqueue Element At Opposite End(queue=w704, element=T7 {"命令"="单个写入", {"starting address"=300, "holding register value"=2}} ("元素")) -> ()  [unwired: 2 in, 3 out]
      }
      event "查看": Value Change {
        n505 = event-data() -> ()  [unwired: 1 in, 6 out]
        n506 = property on="窗格" class="Pane"("Origin"=T1 {"Horizontal"=0, "Vertical"=640} ("原点")) -> ()  [unwired: 2 in, 2 out]
      }
      event "返回": Value Change {
        n507 = event-data() -> ()  [unwired: 1 in, 6 out]
        n508 = property on="窗格" class="Pane"("Origin"=T1 {"Horizontal"=0, "Vertical"=0} ("原点")) -> ()  [unwired: 2 in, 2 out]
      }
    }
  }
  n509 = call-by-ref "?"(reference=w29, error in=w31) -> (reference out=w33:refnum<vi>, error out=w32:errorcluster)  [unwired: 12 in]
  n510 = Open VI Reference(type specifier VI Refnum (for type only)=refnum<vi> refnum, vi path=w20, options=128 ("选项")) -> (vi reference=w18:refnum<vi>, error out=w16:errorcluster)  [unwired: 3 in]
  n511 = call-by-ref "?"(reference=w18, error in=w16) -> (reference out=w14:refnum<vi>, error out=w15:errorcluster)  [unwired: 12 in]
  n512 = Close Reference(reference=w33, error in (no error)=w32) -> ()  [unwired: 1 out]
  n513 = call-by-ref "?"(reference=w9, error in=w11, "CODMn"=w1, "总磷"=w2, "CODCr"=w5, "氨氮"=w3, "总氮"=w4) -> (reference out=w13:refnum<vi>, error out=w12:errorcluster)  [unwired: 7 in]
  n514 = Close Reference(reference=w14, error in (no error)=w15) -> ()  [unwired: 1 out]
  n515 = Close Reference(reference=w13, error in (no error)=w12) -> ()  [unwired: 1 out]
